vi "Auto2备份.vi"() -> ()   [LabVIEW 2020]
uses:
  Global_Variable/Global.vi
  Libraries/S7/S7.lvlib
  Global_Variable/A180648.vi
  <vilib>/ptbypt/NI_PtbyPt.lvlib
  <userlib>/_MGI/1D Array/MGI Average/MGI Average (DBL[][]).vi
panel:
  out "初始角度":dbl
  out "T1-T2_135°":dbl
  out "T1-T2_225°":dbl
  out "T1-T2_315°":dbl
  out "T1-T2_360°":dbl
  out "T1-T2_270°":dbl
  out "T1-T2_180°":dbl
  out "T1-T2_45°":dbl
  out "T1-T2_90°":dbl
  out "初始化 3":bool[](array[boolean])
  out "动优化态前":cluster{dbl[], dbl[]}[](graph)
  in  "initialize 2":bool caption="初始化"
  in  "initialize":bool caption="初始化"
  out "vRES_cCW":cluster{dbl[], dbl[]}
  out "VRES_cW":cluster{dbl[], dbl[]}
  out "初始化 2":bool[](array[boolean])
  in  "选项卡控件":enum32{"工位二程序复检", "工位二动态复检"}(tab)
  out "传感器复检":cluster{dbl[], dbl[]}[](graph)
  out "动优化态":cluster{dbl[], dbl[]}[](graph)
  in  "请启动":bool
  out "Vres_45°":dbl format="%#.6f"
  out "Vres_135°":dbl format="%#.6f"
  out "Vres_225°":dbl format="%#.6f"
  out "Vres_315°":dbl format="%#.6f"
  out "Vres_360°":dbl format="%#.6f"
  out "Vres_270°":dbl format="%#.6f"
  out "Vres_180°":dbl format="%#.6f"
  out "Vres_90°":dbl format="%#.6f"
  out "S_CCw":dbl[](array[numeric]) caption="数据" format="%0.6f"
  out "P_CCw":dbl[](array[numeric]) caption="数据" format="%0.6f"
  out "S_CW":dbl[](array[numeric]) caption="数据" format="%0.6f"
  out "P_CW":dbl[](array[numeric]) caption="数据" format="%0.6f"
  out "T1_CCw":dbl[](array[numeric]) caption="数据" format="%0.2f"
  out "T2_CCw":dbl[](array[numeric]) caption="数据" format="%0.2f"
  out "T2_CW":dbl[](array[numeric]) caption="数据" format="%0.2f"
  out "T1_CW":dbl[](array[numeric]) caption="数据" format="%0.2f"
  out "初始化":bool[](array[boolean])
  out "SENSOR":T1
  in  "判定结果":bool[][](array[boolean])=[[TRUE]]
  in  "STEP":string
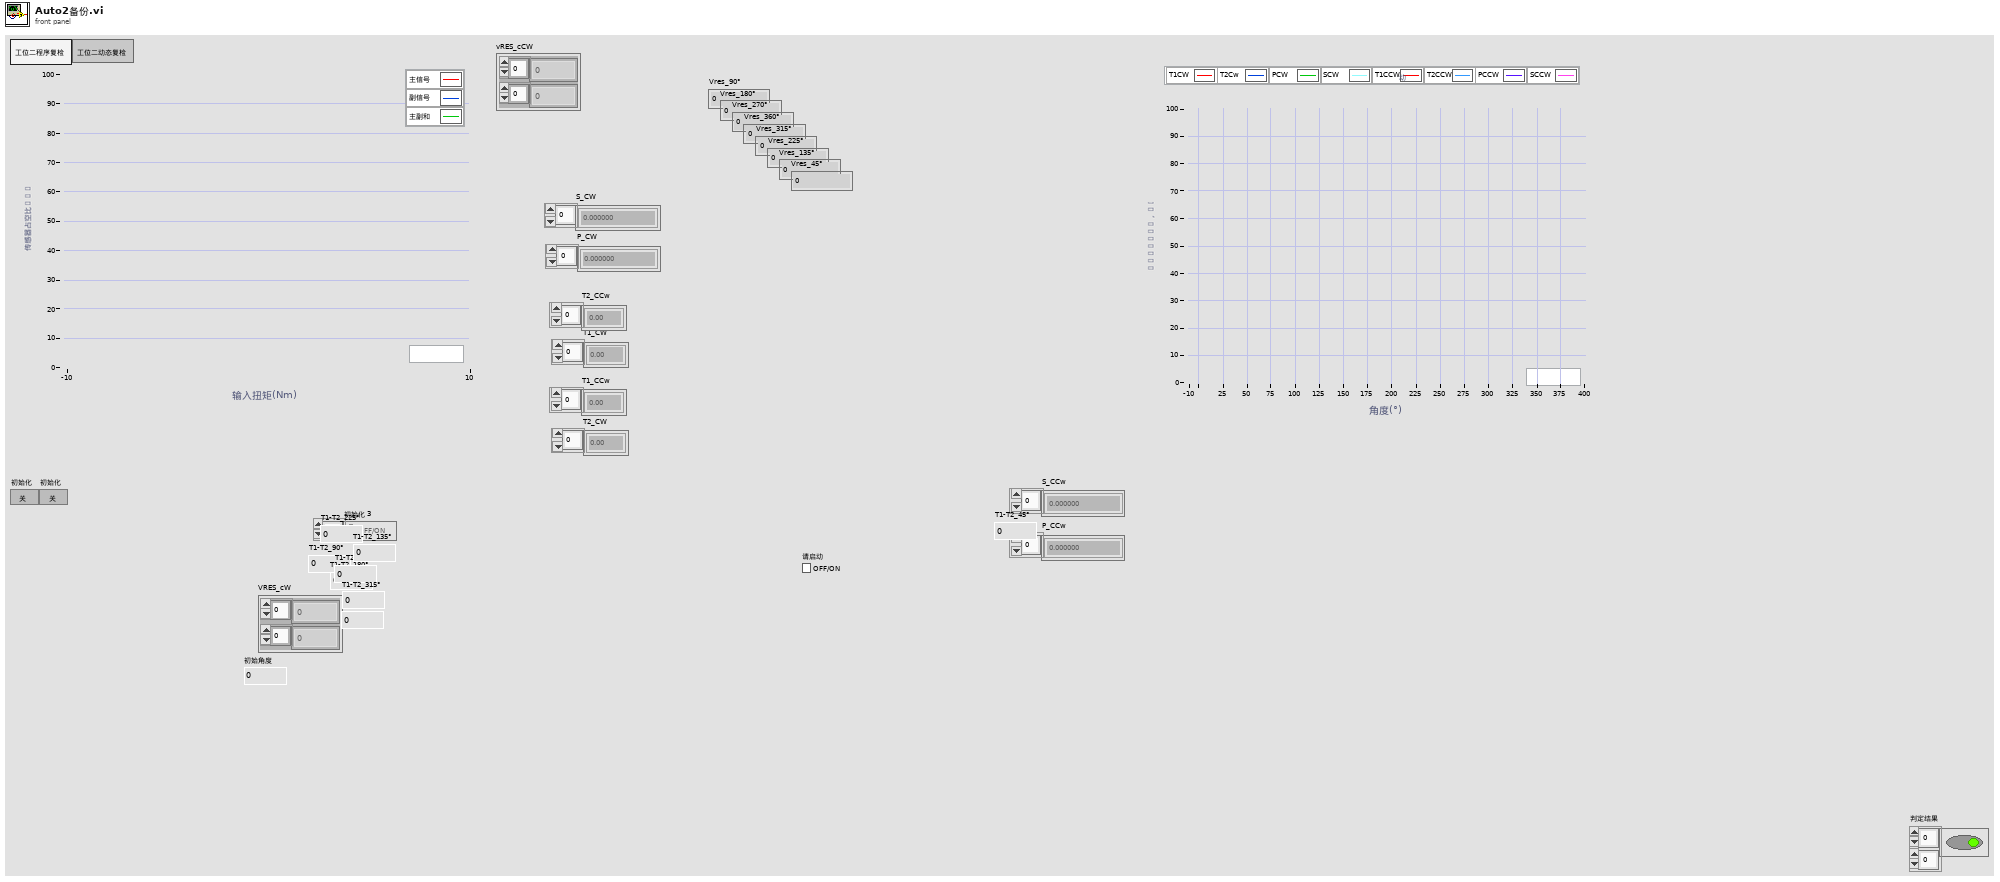
[diagram p1: front panel]
types:
  T1 = cluster{"hSENSOR":i32, "hASIC_T1":i32, "hASIC_T2":i32, "hASIC_P":i32, "hASIC_S":i32}
  T2 = typedef "检测CTR.xctl/检测CTR数据.ctl" = enum16{"Idle", "Runing", "Pass", "Faild", "Skip"}
  T3 = enum32{"Invalid", "Standard", "Closed", "Hidden", "Minimized", "Maximized"}
  T4 = enum16{"Idle", "Runing", "Pass", "Faild", "Skip"}
  T5 = enum16{"open", "replace", "create", "open or create", "replace or create", "replace or create with confirmation"}
  T6 = cluster{"工位一驱动伺服位移":sgl, "工位二驱动伺服位移":sgl, "工位一移载伺服位移":sgl, "工位二移载伺服位移":sgl, "工位一编码器位移":sgl, "工位二编码器位移":sgl, "工位一扭矩":sgl, "工位二扭矩":sgl}
  T7 = cluster{"主副信号和MAX":cluster{"单位":string, "下限":dbl, "上限":dbl}, "主副信号和MIN":cluster{"单位":string, "下限":dbl, "上限":dbl}, "主信号线性误差":cluster{"单位":string, "下限":dbl, "上限":dbl}, "副信号线性误差":cluster{"单位":string, "下限":dbl, "上限":dbl}, "主信号MAX":cluster{"单位":string, "下限":dbl, "上限":dbl}, "主信号MIN":cluster{"单位":string, "下限":dbl, "上限":dbl}, "副信号MAX":cluster{"单位":string, "下限":dbl, "上限":dbl}, "副信号MIN":cluster{"单位":string, "下限":dbl, "上限":dbl}, "中心偏移量":cluster{"单位":string, "下限":dbl, "上限":dbl}, "定点设置":cluster{"单位":string, "下限":dbl, "上限":dbl}, "定点左侧主信号":cluster{"单位":string, "下限":dbl, "上限":dbl}, "定点左侧副信号":cluster{"单位":string, "下限":dbl, "上限":dbl}, "定点右侧主信号":cluster{"单位":string, "下限":dbl, "上限":dbl}, "定点右侧副信号":cluster{"单位":string, "下限":dbl, "上限":dbl}, "监测点1左滞后":cluster{"单位":string, "下限":dbl, "上限":dbl}, "监测点1右滞后":cluster{"单位":string, "下限":dbl, "上限":dbl}, "监测点2左滞后":cluster{"单位":string, "下限":dbl, "上限":dbl}, "监测点2右滞后":cluster{"单位":string, "下限":dbl, "上限":dbl}, "监测点3左滞后":cluster{"单位":string, "下限":dbl, "上限":dbl}, "监测点3右滞后":cluster{"单位":string, "下限":dbl, "上限":dbl}}
  T8 = cluster{"复检速度":dbl, "换向扭矩":dbl, "判定范围下限":dbl, "判定范围上限":dbl, "滞后监测点1":dbl, "滞后监测点2":dbl, "滞后监测点3":dbl}
  T9 = cluster{"动优化态":cluster{dbl[], dbl[]}[], "动优化态前":cluster{dbl[], dbl[]}[], "传感器复检":cluster{dbl[], dbl[]}[]}
  T10 = typedef "lveventtype.ctl" = enum32{"Null", "Timeout", "Annotation Menu Selection", "Annotation Menu Selection?", "App Instance Close", "App Instance Close?", "Autoscale Range Change", "Bookmark Info Change", "Cell Edit", "Cell Edit?", "Cursor Grab", "Cursor Grab?", "Cursor Menu Selection", "Cursor Menu Selection?", "Cursor Move", "Cursor Release", "Data Change", "Direction Change", "Display State Change", "Drag Ended", "Drag Enter", "Drag Leave", "Drag Over", "Drag Source Update", "Drag Starting", "Drag Starting?", "Drop", "Exec State Change", "Key Down", "Key Down?", "Key Repeat", "Key Repeat?", "Key Up", "Listbox Double Click", "Menu Activation?", "Menu Selection (App)", "Menu Selection? (App)", "Menu Selection (User)", "Mouse Down", "Mouse Down?", "Mouse Enter", "Mouse Leave", "Mouse Move", "Mouse Up", "Mouse Wheel", "NI Security User Change (App)", "Pane Size", "Panel Close", "Panel Close?", "Panel Resize", "Plot Attribute Change", "Scale Range Change", "Shortcut Menu Activation?", "Shortcut Menu Selection (App)", "Shortcut Menu Selection? (App)", "Shortcut Menu Selection (User)", "Tree Double Click", "Tree Drag", "Tree Drag?", "Tree Drop", "Tree Drop?", "Tree Item Close", "Tree Item Close?", "Tree Item Open", "Tree Item Open?", "User Event", "Value Change"}
  T11 = typedef "LVPoint32TypeDef.ctl" = cluster{"Horizontal":i32, "Vertical":i32}
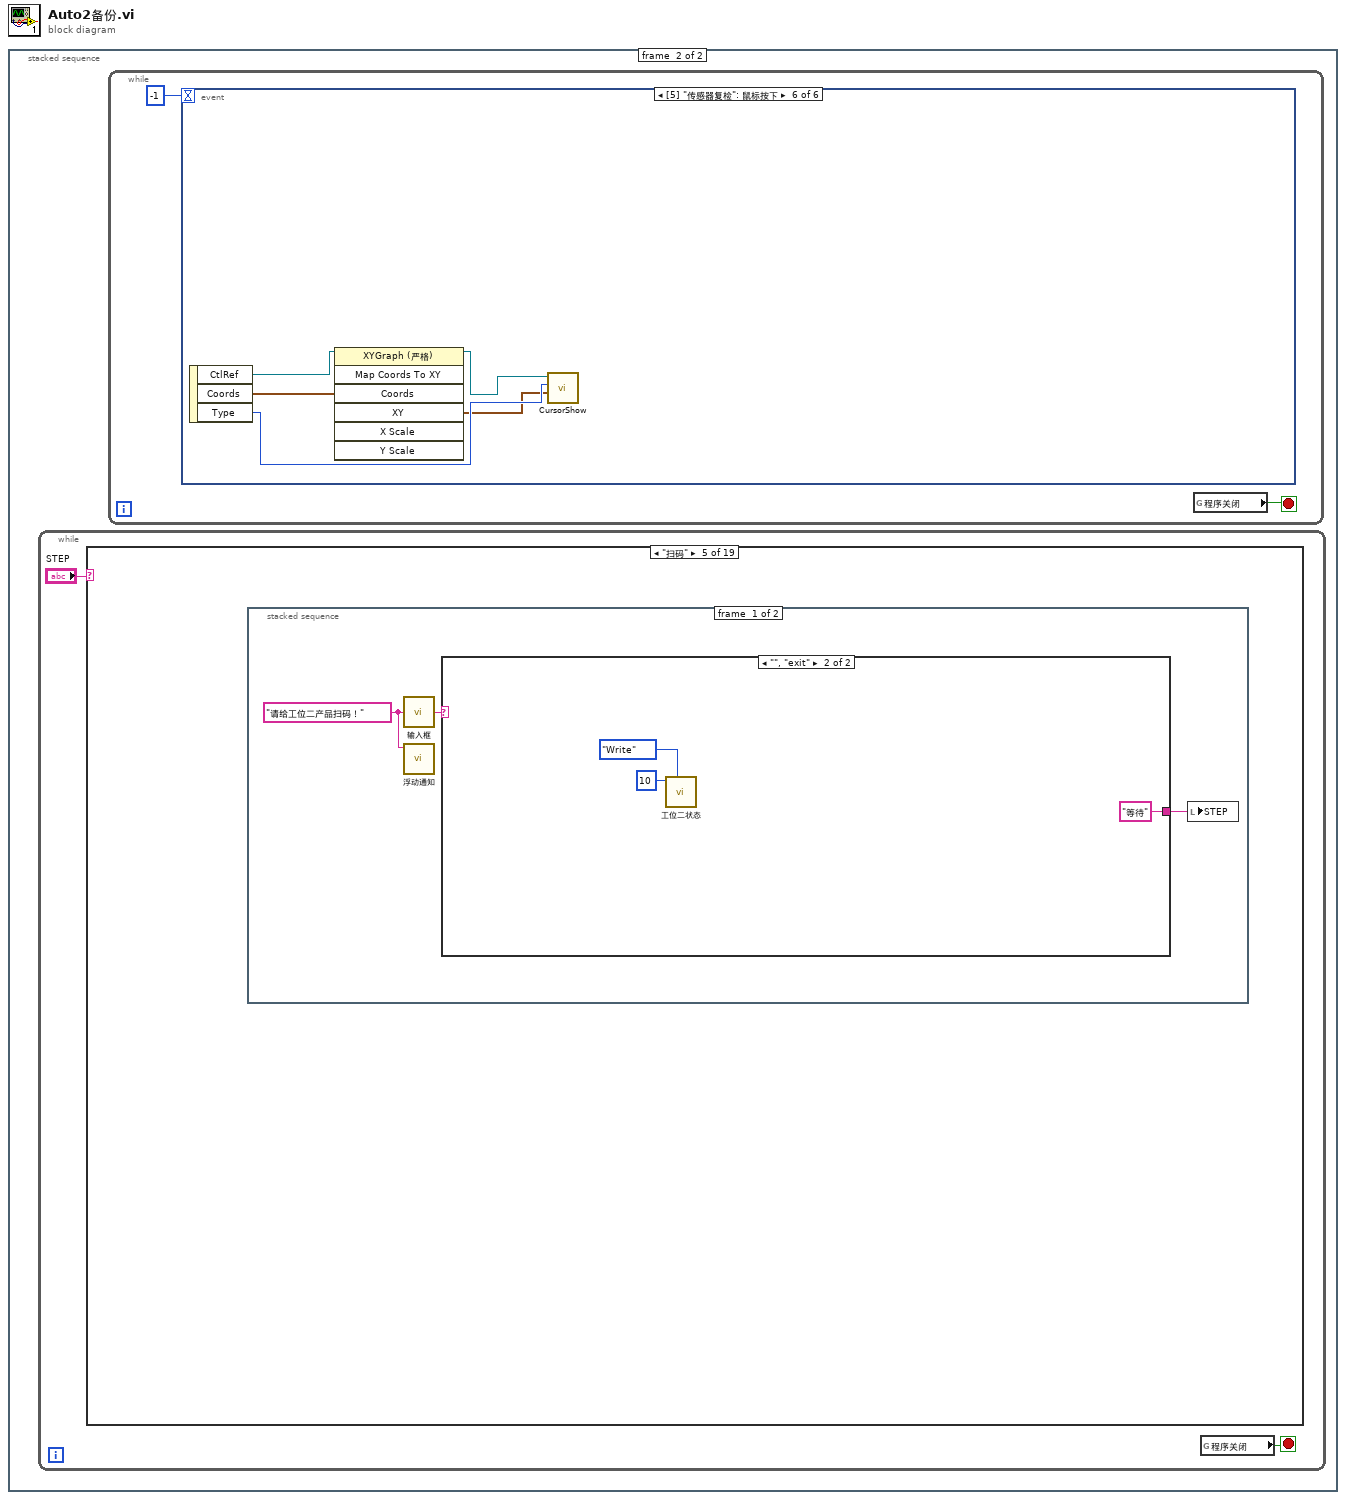
[diagram p0: block diagram]
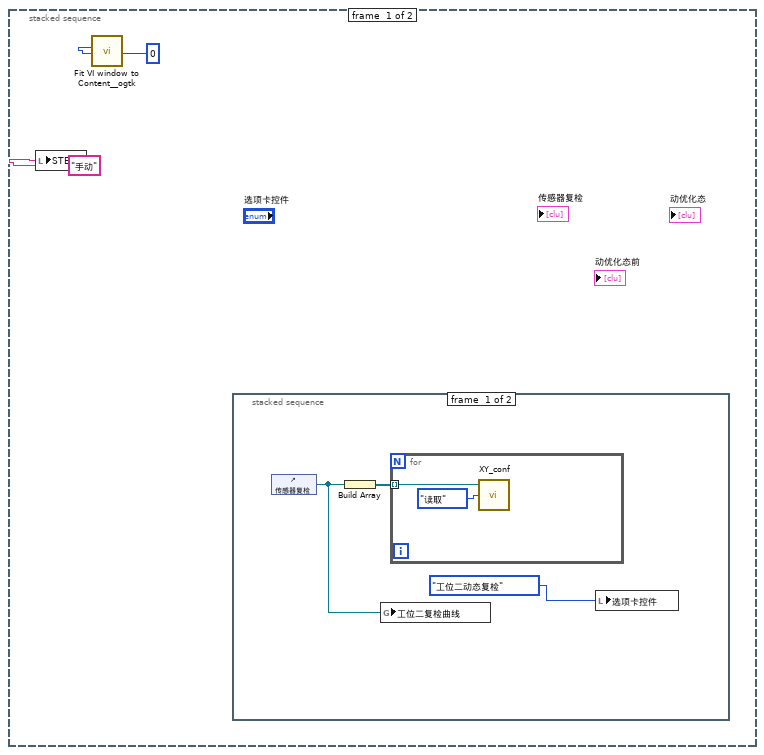
[diagram p2: hidden frame]
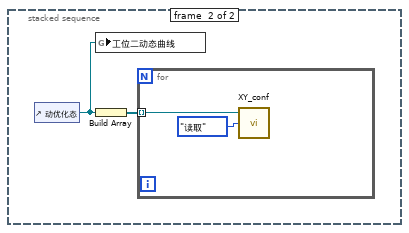
[diagram p3: hidden frame]
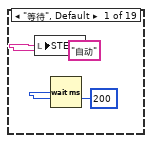
[diagram p4: hidden frame]
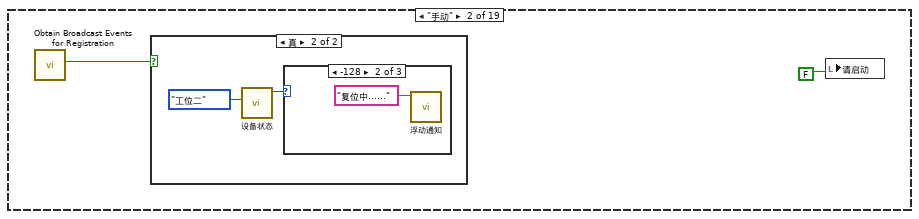
[diagram p5: hidden frame]
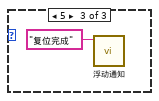
[diagram p8: hidden frame]
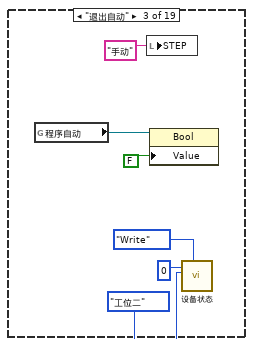
[diagram p9: hidden frame]
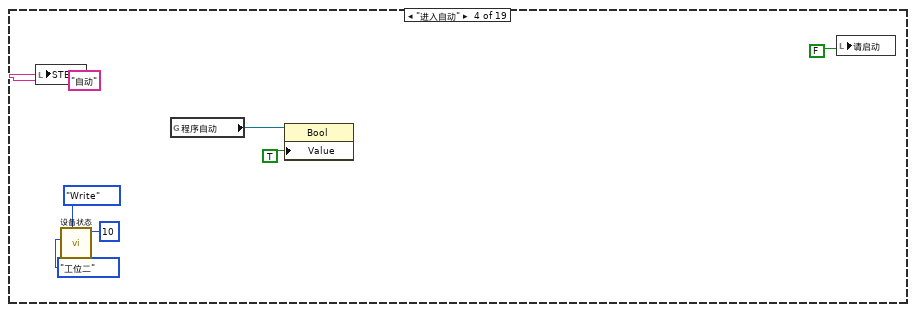
[diagram p10: hidden frame]
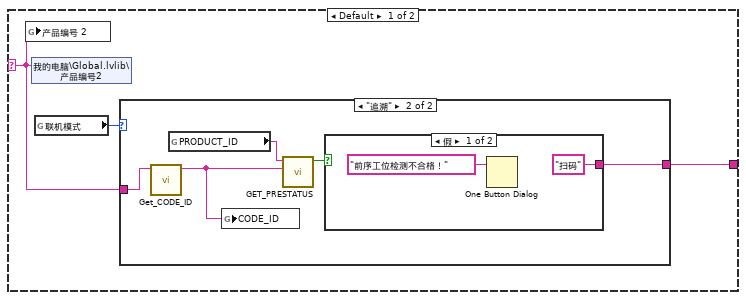
[diagram p11: hidden frame]
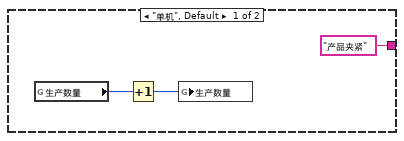
[diagram p12: hidden frame]
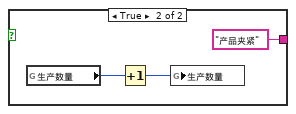
[diagram p13: hidden frame]
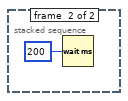
[diagram p14: hidden frame]
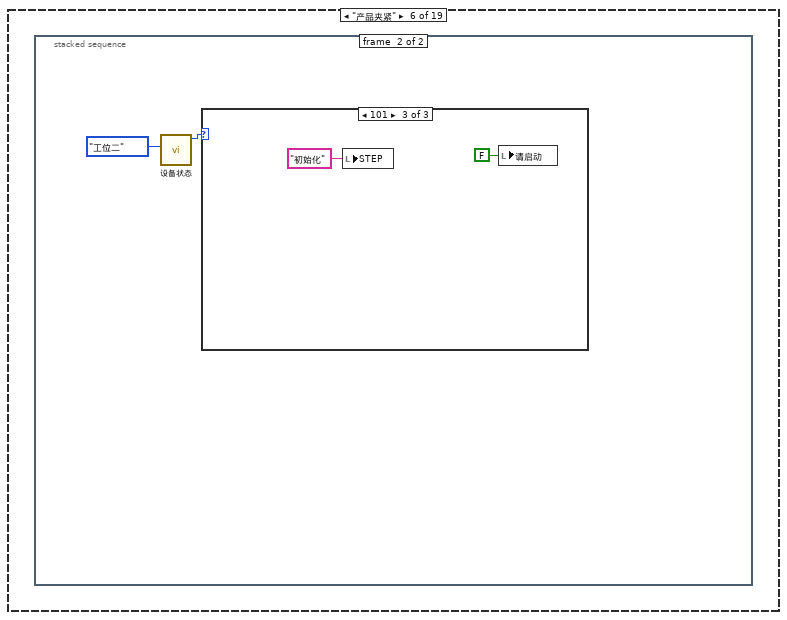
[diagram p15: hidden frame]
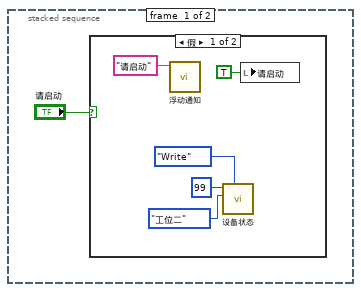
[diagram p16: hidden frame]
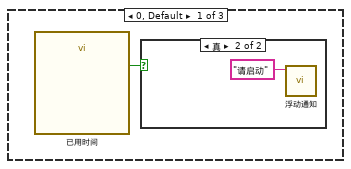
[diagram p18: hidden frame]
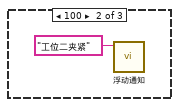
[diagram p20: hidden frame]
diagram:
  n1 = stacked-sequence {
    frame #0 {
      n2 = local write "STEP"("手动" ("STEP")) -> ()
      n3 = call <userlib>:"Fit VI window to Content__ogtk.vi"("border spacing (2 px)"=0) -> ()  [unwired: 5 in, 2 out]
      n4 = stacked-sequence {
        frame #0 {
          n5 = control-ref of="传感器复检"() -> (w4:refnum<vi>)
          n6 = Build Array(w4) -> (w5:refnum<vi>[])
          n7 = global write "A180648.vi" "工位二复检曲线"(w4) -> ()
          n8 = for {
            tunnel: w5 -> [w6] mode=indexing
            n9 = call "XY_conf.vi"("方式"=enum16{"写入", "读取"}."读取", "XY图引用"=w6) -> ()  [unwired: 3 in, 1 out]
          }
          n10 = local write "选项卡控件"(enum32{"工位二程序复检", "工位二动态复检"}."工位二动态复检" ("选项卡控件")) -> ()
        }
        frame #1 {
          n11 = control-ref of="动优化态"() -> (w9:refnum<vi>)
          n12 = global write "A180648.vi" "工位二动态曲线"(w9) -> ()
          n13 = Build Array(w9) -> (w8:refnum<vi>[])
          n14 = for {
            tunnel: w8 -> [w10] mode=indexing
            n15 = call "XY_conf.vi"("方式"=enum16{"写入", "读取"}."读取", "XY图引用"=w10) -> ()  [unwired: 3 in, 1 out]
          }
        }
      }
    }
    frame #1 {
      n16 = while {
        stop <- w13 stop-if-true
        n17 = case shown="\"扫码\"" "STEP" {
          frame "等待", Default {
            n18 = local write "STEP"("自动" ("STEP")) -> ()
            n19 = Wait (ms)(milliseconds to wait=u32 200 ("等待时间（毫秒）")) -> ()  [unwired: 1 out]
          }
          frame "手动" {
            n20 = call "Obtain Broadcast Events for Registration.vi"() -> ("Already running?"=w17:bool)  [unwired: 9 in, 2 out]
            n21 = case shown="真" w17 {
              frame False {
              }
              frame True {
                n22 = call "设备状态.vi"("工位"=enum16{"工位一", "工位二"}."工位二") -> ("Status_Read"=w19:i16)  [unwired: 10 in]
                n23 = case shown="-128" w19 {
                  frame 0, Default {
                  }
                  frame -128 {
                    n24 = call "浮动通知.vi"("通知内容"="复位中……" ("Status")) -> ()  [unwired: 11 in]
                  }
                  frame 5 {
                    n25 = call "浮动通知.vi"("通知内容"="复位完成" ("Status")) -> ()  [unwired: 11 in]
                  }
                }
              }
            }
            n26 = local write "请启动"(FALSE ("请启动")) -> ()
          }
          frame "退出自动" {
            n27 = global read "Global.vi" "程序自动"() -> (w24:refnum<vi>)
            n28 = local write "STEP"("手动" ("STEP")) -> ()
            n29 = property class="Bool"(reference=w24, "Value"=FALSE) -> ()  [unwired: 1 in, 2 out]
            n30 = call "设备状态.vi"("枚举"=enum16{"Read", "Write"}."Write", "工位"=enum16{"工位一", "工位二"}."工位二", "Status_Write"=i16 0) -> ()  [unwired: 8 in, 1 out]
          }
          frame "进入自动" {
            n31 = local write "STEP"("自动" ("STEP")) -> ()
            n32 = call "设备状态.vi"("枚举"=enum16{"Read", "Write"}."Write", "工位"=enum16{"工位一", "工位二"}."工位二", "Status_Write"=i16 10) -> ()  [unwired: 8 in, 1 out]
            n33 = global read "Global.vi" "程序自动"() -> (w33:refnum<vi>)
            n34 = property class="Bool"(reference=w33, "Value"=TRUE) -> ()  [unwired: 1 in, 2 out]
            n35 = local write "请启动"(FALSE ("请启动")) -> ()
          }
          frame "扫码" {
            n36 = stacked-sequence {
              frame #0 {
                w36 = "请给工位二产品扫码！" ("提示信息")
                n37 = call "输入框.vi"("提示信息"=w36) -> ("条形码输出"=w37:string)
                n38 = call "浮动通知.vi"("通知内容"=w36) -> ()  [unwired: 11 in]
                n39 = case shown="\"\", \"exit\"" w37 {
                  selector: w37 -> [w38 _]
                  tunnel: [w40 "等待" ("State(s) in Front (\"\")")] -> w35
                  frame Default {
                    n40 = global write "Global.vi" "产品编号 2"(w38) -> ()
                    n41 = shared-variable "我的电脑\\Global.lvlib\\产品编号2"(w38) -> ()  [unwired: 1 in, 1 out]
                    n42 = global read "Global.vi" "联机模式"() -> (w39:enum16{"单机", "追溯"})
                    n43 = case shown="\"追溯\"" w39 {
                      tunnel: ["产品夹紧" ("State(s) in Front (\"\")") w48] -> w40
                      tunnel: w38 -> [_ w45]
                      frame "单机", Default {
                        n44 = global read "Global.vi" "生产数量"() -> (w41:i32)
                        n45 = Increment(x=w41) -> (x+1=w42:i32)
                        n46 = global write "Global.vi" "生产数量"(w42) -> ()
                      }
                      frame "追溯" {
                        n47 = call "Get_CODE_ID.vi"("CODE_MAIN"=w45) -> ("CODE_ID"=w44:string)  [unwired: 10 in]
                        n48 = global read "追溯Global.vi" "PRODUCT_ID"() -> (w47:string)
                        n49 = global write "追溯Global.vi" "CODE_ID"(w44) -> ()
                        n50 = call "GET_PRESTATUS.vi"("CODE_ID"=w44, "PRODUCT_ID"=w47) -> ("OK?"=w46:bool)  [unwired: 9 in]
                        n51 = case shown="假" w46 {
                          tunnel: ["扫码" ("State(s) in Front (\"\")") "产品夹紧" ("State(s) in Front (\"\")")] -> w48
                          frame False {
                            n52 = One Button Dialog(message="前序工位检测不合格！" ("消息")) -> ()  [unwired: 1 in, 1 out]
                          }
                          frame True {
                            n53 = global read "Global.vi" "生产数量"() -> (w51:i32)
                            n54 = Increment(x=w51) -> (x+1=w52:i32)
                            n55 = global write "Global.vi" "生产数量"(w52) -> ()
                          }
                        }
                      }
                    }
                  }
                  frame "", "exit" {
                    n56 = call "工位二状态.vi"("枚举"=enum16{"Read", "Write"}."Write", "Status_Write"=i16 10) -> ()  [unwired: 9 in, 1 out]
                  }
                }
                n57 = local write "STEP"(w35) -> ()
              }
              frame #1 {
                n58 = Wait (ms)(milliseconds to wait=u32 200 ("等待时间（毫秒）")) -> ()  [unwired: 1 out]
              }
            }
          }
          frame "产品夹紧" {
            n59 = stacked-sequence {
              frame #0 {
                n60 = case shown="假" "请启动" {
                  frame False {
                    n61 = call "浮动通知.vi"("通知内容"="请启动" ("Status")) -> ()  [unwired: 11 in]
                    n62 = call "设备状态.vi"("枚举"=enum16{"Read", "Write"}."Write", "工位"=enum16{"工位一", "工位二"}."工位二", "Status_Write"=i16 99) -> ()  [unwired: 8 in, 1 out]
                    n63 = local write "请启动"(TRUE ("请启动")) -> ()
                  }
                  frame True {
                  }
                }
              }
              frame #1 {
                n64 = call "设备状态.vi"("工位"=enum16{"工位一", "工位二"}."工位二") -> ("Status_Read"=w64:i16)  [unwired: 10 in]
                n65 = case shown="101" w64 {
                  frame 0, Default {
                    n66 = call "已用时间"() -> ("Time has Elapsed"=w66:bool)  [unwired: 12 in, 7 out]
                    n67 = case shown="真" w66 {
                      frame False {
                      }
                      frame True {
                        n68 = call "浮动通知.vi"("通知内容"="请启动" ("Status")) -> ()  [unwired: 11 in]
                      }
                    }
                  }
                  frame 100 {
                    n69 = call "浮动通知.vi"("通知内容"="工位二夹紧" ("Status")) -> ()  [unwired: 11 in]
                  }
                  frame 101 {
                    n70 = local write "STEP"("初始化") -> ()
                    n71 = local write "请启动"(FALSE ("请启动")) -> ()
                  }
                }
              }
            }
          }
          frame "套输入轴" {
            n72 = global read "Global.vi" "复检2引用句柄"() -> (w80)
            n73 = global read "Global.vi" "动态优化 2"() -> (w77)
            n74 = property class="检测CTR"(reference=w77) -> ("Value"=w78:variant)  [unwired: 1 in, 2 out]
            n75 = property class="检测CTR"(reference=w80) -> ("Value"=w79:variant)  [unwired: 1 in, 2 out]
            n76 = Variant To Data(type=检测CTR数据."Idle" ("Data"), Variant=w78) -> (data=w76:T2)  [unwired: 1 in, 1 out]
            n77 = Variant To Data(type=检测CTR数据."Idle" ("Data"), Variant=w79) -> (data=w81:T2)  [unwired: 1 in, 1 out]
            n78 = Equal?(x=w76, y=检测CTR数据."Skip" ("Data")) -> (x = y?=w82:bool)
            n79 = Equal?(x=w81, y=检测CTR数据."Skip" ("Data")) -> (x = y?=w83:bool)
            n80 = And(x=w82, y=w83) -> (x .and. y?=w71:bool)
            n81 = case shown="假" w71 {
              frame False {
                n82 = stacked-sequence {
                  frame #0 {
                    n83 = call "浮动通知.vi"("通知内容"="工位二产品套输入轴" ("Status")) -> ()  [unwired: 11 in]
                    n84 = call "设备状态.vi"("枚举"=enum16{"Read", "Write"}."Write", "工位"=enum16{"工位一", "工位二"}."工位二", "Status_Write"=i16 112) -> ()  [unwired: 8 in, 1 out]
                    n85 = vi-ref "T1T2占空比2.vi"() -> (w87:refnum<vi>)
                    n86 = call "CallVI.vi"("VI引用"=w87, "状态"=T3."Hidden") -> ()  [unwired: 12 in, 2 out]
                    n87 = vi-ref "PS采集2.vi"() -> (w84:refnum<vi>)
                    n88 = call "CallVI.vi"("VI引用"=w84, "状态"=T3."Hidden") -> ()  [unwired: 12 in, 2 out]
                  }
                  frame #1 {
                    n89 = while {
                      stop <- w92 stop-if-true
                      n90 = call "设备状态.vi"("工位"=enum16{"工位一", "工位二"}."工位二") -> ("Status_Read"=w93:i16)  [unwired: 10 in]
                      n91 = case shown="113" w93 {
                        tunnel: [w95 TRUE] -> w92
                        frame 0, Default {
                          n92 = call "套输入轴时间"() -> ("Time has Elapsed"=w96:bool)  [unwired: 12 in, 7 out]
                          n93 = case shown="真" w96 {
                            tunnel: [FALSE TRUE] -> w95
                            frame False {
                            }
                            frame True {
                              n94 = call "浮动通知.vi"("通知内容"="工位二产品套输入轴超时" ("Status")) -> ()  [unwired: 11 in]
                            }
                          }
                        }
                        frame 113 {
                          n95 = local write "STEP"("动态优化") -> ()
                        }
                      }
                    }
                  }
                }
              }
              frame True {
                n96 = local write "STEP"("程序固化" ("STEP")) -> ()
              }
            }
          }
          frame "套输出轴" {
            n97 = global read "Global.vi" "复检2引用句柄"() -> (w107)
            n98 = property class="检测CTR"(reference=w107) -> ("Value"=w106:variant)  [unwired: 1 in, 2 out]
            n99 = Variant To Data(type=检测CTR数据."Idle" ("Data"), Variant=w106) -> (data=w108:T2)  [unwired: 1 in, 1 out]
            n100 = Equal?(x=w108, y=检测CTR数据."Skip" ("Data")) -> (x = y?=w103:bool)
            n101 = case shown="假" w103 {
              frame False {
                n102 = stacked-sequence {
                  frame #0 {
                    n103 = call "设备状态.vi"("枚举"=enum16{"Read", "Write"}."Write", "工位"=enum16{"工位一", "工位二"}."工位一", "Status_Write"=i16 108) -> ()  [unwired: 8 in, 1 out]
                    n104 = call "浮动通知.vi"("通知内容"="工位一产品套输出轴" ("Status")) -> ()  [unwired: 11 in]
                  }
                  frame #1 {
                    n105 = while {
                      stop <- w113 stop-if-true
                      n106 = call "设备状态.vi"("工位"=enum16{"工位一", "工位二"}."工位二") -> ("Status_Read"=w114:i16)  [unwired: 10 in]
                      n107 = case shown="109" w114 {
                        tunnel: [w116 TRUE] -> w113
                        frame 0, Default {
                          n108 = call "套输出轴时间"() -> ("Time has Elapsed"=w117:bool)  [unwired: 12 in, 7 out]
                          n109 = case shown="真" w117 {
                            tunnel: [FALSE TRUE] -> w116
                            frame False {
                            }
                            frame True {
                              n110 = call "浮动通知.vi"("通知内容"="工位二产品套输出轴超时" ("Status")) -> ()  [unwired: 11 in]
                            }
                          }
                        }
                        frame 109 {
                          n111 = call "传感器数据.vi"() -> ("传感器读数"=w122:T6)  [unwired: 11 in]
                          n112 = local write "STEP"("程序复检") -> ()
                          n113 = Unbundle By Name(w122) -> ("工位二驱动伺服位移"=→"初始角度":sgl)
                        }
                      }
                    }
                  }
                }
              }
              frame True {
                n114 = local write "STEP"("程序固化" ("STEP")) -> ()
              }
            }
          }
          frame "初始化" {
            n115 = stacked-sequence {
              frame #0 {
                w128 = cluster{dbl[], dbl[]} {[], []} ("vRES_cCW")
                n116 = disable-structure shown="禁用" {
                  frame Disabled {
                    n117 = global write "Global.vi" "计时开始"(TRUE ("计时开始")) -> ()
                  }
                  frame Enabled {
                  }
                }
                n118 = global write "Global.vi" "IO_Stop"(TRUE ("IO_Stop")) -> ()
                n119 = global write "Global.vi" "工位二占空比采集"(FALSE ("工位二占空比采集")) -> ()
                n120 = global write "Global.vi" "P/S采集 2"(FALSE ("工位二占空比采集")) -> ()
                n121 = local write "判定结果"(bool[][] [] ("判定结果")) -> ()
                n122 = global write "Global.vi" "动态优化完成"(FALSE ("动态优化完成")) -> ()
                n123 = local write "vRES_cCW"(w128) -> ()
                n124 = local write "VRES_cW"(w128) -> ()
                n125 = local write "选项卡控件"(enum32{"工位二程序复检", "工位二动态复检"}."工位二动态复检" ("选项卡控件")) -> ()
              }
              frame #1 {
                w139 = dbl[] [] ("S_CCw")
                w140 = dbl[] [] ("T1_cw")
                n126 = local write "T1_CW"(w140) -> ()
                n127 = local write "T2_CW"(w140) -> ()
                n128 = local write "P_CW"(w140) -> ()
                n129 = local write "P_CCw"(w140) -> ()
                n130 = for {
                  N: 12 -> [_]
                  tunnel: [cluster{dbl[], dbl[]} {[], []}] -> w138 mode=indexing
                }
                n131 = local write "传感器复检"(w138) -> ()
                n132 = local write "S_CCw"(w139) -> ()
                n133 = local write "S_CW"(w139) -> ()
                n134 = local write "T1_CCw"(w139) -> ()
                n135 = local write "T2_CCw"(w139) -> ()
                n136 = for {
                  N: 8 -> [_]
                  tunnel: [cluster{dbl[], dbl[]} {[], []}] -> w136 mode=indexing
                }
                n137 = for {
                  N: 8 -> [_]
                  tunnel: [cluster{dbl[], dbl[]} {[], []}] -> w135 mode=indexing
                }
                n138 = local write "动优化态前"(w135) -> ()
                n139 = local write "动优化态"(w136) -> ()
              }
              frame #2 {
                n140 = global read "Global.vi" "Result 2"() -> (w156)
                n141 = property class="Tbl"(reference=w156, "Value"=string[][] []) -> (reference out=w157:refnum<vi>, error out=w158:errorcluster)  [unwired: 1 in]
                n142 = property class="Tbl"(reference=w157, error in=w158, "Row Headers[]"=string[] [] ("列首字符串[]")) -> ()  [unwired: 2 out]
                n143 = Initialize Array(TRUE, 12 ("维数大小")) -> (→"初始化":bool[])
                n144 = Initialize Array(TRUE, 8 ("维数大小")) -> (→"初始化 2":bool[])
                n145 = Initialize Array(TRUE, 8 ("维数大小")) -> (→"初始化 3":bool[])
              }
              frame #3 {
                n146 = global read "Global.vi" "静态标定2引用句柄"() -> (w163)
                n147 = global read "Global.vi" "程序固化2引用句柄"() -> (w162)
                n148 = global read "Global.vi" "复检2引用句柄"() -> (w161)
                n149 = global read "Global.vi" "动态优化 2"() -> (w159)
                n150 = Build Array(w163, w162, w161, w159) -> (w160:void[])
                n151 = for {
                  tunnel: w160 -> [w173] mode=indexing
                  n152 = property class="检测CTR"(reference=w173) -> (reference out=w172:refnum<vi>, "Value"=w171:variant)  [unwired: 1 in, 1 out]
                  n153 = Variant To Data(type=检测CTR数据."Idle" ("Data"), Variant=w171) -> (data=w169:T2)  [unwired: 1 in, 1 out]
                  n154 = Equal?(x=w169, y=检测CTR数据."Skip" ("Data")) -> (x = y?=w167:bool)
                  n155 = Select(t=检测CTR数据."Skip" ("Data"), s=w167, f=检测CTR数据."Idle" ("Data")) -> (s? t:f=w164:T2)
                  n156 = property class="检测CTR"(reference=w172, "Value"=w164) -> ()  [unwired: 1 in, 2 out]
                }
              }
              frame #4 {
                n157 = local write "STEP"("静态标定" ("STEP")) -> ()
              }
            }
          }
          frame "静态标定" {
            n158 = global read "Global.vi" "静态标定2引用句柄"() -> (w179)
            n159 = property class="检测CTR"(reference=w179) -> ("Value"=w178:variant)  [unwired: 1 in, 2 out]
            n160 = Variant To Data(type=检测CTR数据."Idle" ("Data"), Variant=w178) -> (data=w180:T2)  [unwired: 1 in, 1 out]
            n161 = Equal?(x=w180, y=检测CTR数据."Skip" ("Data")) -> (x = y?=w175:bool)
            n162 = case shown="假" w175 {
              frame False {
                n163 = stacked-sequence {
                  tunnel: [_ _ w189] -> w181
                  frame #0 {
                    n164 = call "InitPGI.vi"("DeviceNumber"=2) -> ("SENSOR"=w183:T1, "error out"=w184:errorcluster)  [unwired: 13 in]
                    "SENSOR" <- w183
                    n165 = call "InitProduct.vi"("SENSOR"=w183, "error in (no error)"=w184) -> ()  [unwired: 12 in, 2 out]
                  }
                  frame #1 {
                    n166 = global read "Global.vi" "静态标定2引用句柄"() -> (w186)
                    n167 = call "浮动通知.vi"("通知内容"="静态标定" ("Status")) -> ()  [unwired: 11 in]
                    n168 = property class="检测CTR"(reference=w186, "Value"=T4."Runing" ("值")) -> ()  [unwired: 1 in, 2 out]
                  }
                  frame #2 {
                    n169 = flat-sequence {
                      frame #0 {
                        n170 = call "采集切换2.vi"("切换"=TRUE) -> ()  [unwired: 10 in, 1 out]
                      }
                      frame #1 {
                        n171 = call "Wait1.vi"("Wait（150ms）"=u32 500) -> ()  [unwired: 2 in, 1 out]
                      }
                      frame #2 {
                        n172 = call "采集切换2.vi"("切换"=FALSE) -> ()  [unwired: 10 in, 1 out]
                      }
                      frame #3 {
                        n173 = call "采集切换2.vi"("切换"=TRUE) -> ()  [unwired: 10 in, 1 out]
                      }
                      frame #4 {
                        n174 = call "采集切换2.vi"("切换"=FALSE) -> ()  [unwired: 10 in, 1 out]
                      }
                      frame #5 {
                        n175 = call "采集切换2.vi"("切换"=TRUE) -> ()  [unwired: 10 in, 1 out]
                      }
                      frame #6 {
                        n176 = call "Wait1.vi"("Wait（150ms）"=u32 200) -> ()  [unwired: 2 in, 1 out]
                      }
                      frame #7 {
                        n177 = call "采集切换2.vi"("切换"=FALSE) -> ()  [unwired: 10 in, 1 out]
                      }
                    }
                    n178 = local read "SENSOR"() -> (w190:T1)
                    n179 = call "StaticCalibration2备份.vi"("SENSOR"=w190) -> ("OK"=w188:bool)  [unwired: 6 in, 8 out]
                    n180 = case shown="真" w188 {
                      tunnel: [w199 "套输入轴"] -> w189
                      frame False {
                        n181 = global read "Global.vi" "静态标定2引用句柄"() -> (w207)
                        n182 = property class="检测CTR"(reference=w207, "Value"=T4."Faild" ("值")) -> ()  [unwired: 1 in, 2 out]
                        n183 = Two Button Dialog(message="静态标定失败\n建议旋转传感器后重新标定\n是否重新标定？" ("消息"), 1:"否" ("F按钮名称（“取消”）"), 2:"是" ("T按钮名称（“确定”）")) -> (T button?=w202:bool)
                        n184 = Select(t="初始化" ("T按钮名称（“确定”）"), s=w202, f="不合格" ("F按钮名称（“取消”）")) -> (s? t:f=w199:string)
                      }
                      frame True {
                        n185 = global read "Global.vi" "静态标定引用句柄"() -> (w212:refnum<vi>)
                        n186 = local read "判定结果"() -> (w208:bool[][])
                        n187 = Build Array (concatenate)(w208, bool[][] [[TRUE, TRUE]] ("判定结果")) -> (w210:bool[][])
                        n188 = local write "判定结果"(w210) -> ()
                        n189 = property class="检测CTR"(reference=w212, "Value"=T4."Pass" ("值")) -> ()  [unwired: 1 in, 2 out]
                      }
                    }
                  }
                }
                n190 = local write "STEP"(w181) -> ()
              }
              frame True {
                n191 = local write "STEP"("套输入轴") -> ()
                n192 = local read "判定结果"() -> (w214:bool[][])
                n193 = Build Array (concatenate)(w214, bool[][] [[FALSE, TRUE], [FALSE, TRUE]] ("判定结果")) -> (w216:bool[][])
                n194 = local write "判定结果"(w216) -> ()
              }
            }
          }
          frame "动态优化" {
            n195 = global read "Global.vi" "动态优化 2"() -> (w222)
            n196 = property class="检测CTR"(reference=w222) -> ("Value"=w221:variant)  [unwired: 1 in, 2 out]
            n197 = Variant To Data(type=检测CTR数据."Idle" ("Data"), Variant=w221) -> (data=w223:T2)  [unwired: 1 in, 1 out]
            n198 = Equal?(x=w223, y=检测CTR数据."Skip" ("Data")) -> (x = y?=w218:bool)
            n199 = case shown="假" w218 {
              frame False {
                n200 = stacked-sequence {
                  frame #0 {
                    n201 = global read "Global.vi" "动态优化 2"() -> (w226)
                    n202 = call "浮动通知.vi"("通知内容"="动态优化" ("Status")) -> ()  [unwired: 11 in]
                    n203 = property class="检测CTR"(reference=w226, "Value"=T4."Runing" ("值")) -> ()  [unwired: 1 in, 2 out]
                  }
                  frame #1 {
                    n204 = global read "Global.vi" "跳过优化"() -> (w228:bool)
                    n205 = case shown="真" w228 {
                      selector: w228 -> [_ w235]
                      tunnel: ["自动" w233] -> w227
                      frame False {
                        n206 = call "设备状态.vi"("枚举"=enum16{"Read", "Write"}."Write", "工位"=enum16{"工位一", "工位二"}."工位二", "Status_Write"=i16 505) -> ()  [unwired: 8 in, 1 out]
                      }
                      frame True {
                        n207 = global read "Global.vi" "动态优化复测"() -> (w234:bool)
                        n208 = global write "Global.vi" "动态优化完成"(w235) -> ()
                        n209 = case shown="假" w234 {
                          tunnel: [w236 "自动"] -> w233
                          frame False {
                            n210 = global read "Global.vi" "8点复测"() -> (w237:bool)
                            n211 = case shown="假" w237 {
                              tunnel: ["复测判定" "复测"] -> w236
                              frame False {
                              }
                              frame True {
                              }
                            }
                          }
                          frame True {
                            n212 = call "设备状态.vi"("枚举"=enum16{"Read", "Write"}."Write", "工位"=enum16{"工位一", "工位二"}."工位一", "Status_Write"=i16 505) -> ()  [unwired: 8 in, 1 out]
                          }
                        }
                      }
                    }
                    n213 = local write "STEP"(w227) -> ()
                  }
                }
              }
              frame True {
                n214 = local write "STEP"("套输出轴") -> ()
                n215 = local read "判定结果"() -> (w245:bool[][])
                n216 = Build Array (concatenate)(w245, bool[][] [[FALSE, TRUE]] ("判定结果")) -> (w246:bool[][])
                n217 = local write "判定结果"(w246) -> ()
              }
            }
          }
          frame "复测" {
            n218 = stacked-sequence {
              frame #0 {
                n219 = Wait (ms)(milliseconds to wait=u32 300 ("等待时间（毫秒）")) -> ()  [unwired: 1 out]
              }
              frame #1 {
                n220 = local write "STEP"("自动") -> ()
                n221 = call "浮动通知.vi"("通知内容"="复测" ("Status")) -> ()  [unwired: 11 in]
                n222 = call "设备状态.vi"("枚举"=enum16{"Read", "Write"}."Write", "工位"=enum16{"工位一", "工位二"}."工位二", "Status_Write"=i16 510) -> ()  [unwired: 8 in, 1 out]
              }
            }
          }
          frame "复测判定" {
            n223 = local read "Vres_90°"() -> (w273:dbl)
            n224 = local read "Vres_180°"() -> (w272:dbl)
            n225 = local read "Vres_270°"() -> (w271:dbl)
            n226 = local read "Vres_360°"() -> (w270:dbl)
            n227 = local read "Vres_315°"() -> (w265:dbl)
            n228 = local read "Vres_225°"() -> (w264:dbl)
            n229 = local read "Vres_135°"() -> (w263:dbl)
            n230 = local read "Vres_45°"() -> (w269:dbl)
            n231 = local read "T1-T2_90°"() -> (w262:dbl)
            n232 = local read "T1-T2_180°"() -> (w261:dbl)
            n233 = local read "T1-T2_270°"() -> (w260:dbl)
            n234 = local read "T1-T2_360°"() -> (w256:dbl)
            n235 = local read "T1-T2_315°"() -> (w257:dbl)
            n236 = local read "T1-T2_225°"() -> (w258:dbl)
            n237 = local read "T1-T2_135°"() -> (w259:dbl)
            n238 = local read "T1-T2_45°"() -> (w268:dbl)
            n239 = Build Array(w273, w272, w271, w270, w265, w264, w263, w269) -> (w254:dbl[])
            n240 = Build Array(w262, w261, w260, w256, w257, w258, w259, w268) -> (w267:dbl[])
            n241 = Absolute Value(x=w267) -> (abs(x)=w266:dbl[])
            n242 = disable-structure shown="禁用" {
              frame Disabled {
                n243 = Two Button Dialog(message="复测失败\n请选择是否继续？" ("消息"), 1:"否" ("F按钮名称（“取消”）"), 2:"是" ("T按钮名称（“确定”）")) -> ()  [unwired: 1 out]
                n244 = case shown="真" {
                  selector: _ -> [_ _]
                  frame False {
                  }
                  frame True {
                    n245 = local write "STEP"("套输出轴" ("T按钮名称（“确定”）")) -> ()
                  }
                }
              }
              frame Enabled {
              }
            }
            n246 = call "动态优化复测判定.vi"("T1-T2"=w266, "Vres"=w254) -> ("结果1"=w255:bool)  [unwired: 9 in]
            n247 = case shown="真" w255 {
              frame False {
                w280 = enum16{"Read", "Write"}."Write" ("枚举")
                w279 = enum16{"工位一", "工位二"}."工位二" ("工位")
                n248 = global read "Global.vi" "动态优化 2"() -> (w287)
                n249 = local read "判定结果"() -> (w283:bool[][])
                n250 = Build Array (concatenate)(w283, bool[][] [[TRUE, FALSE]] ("判定结果")) -> (w284:bool[][])
                n251 = local write "判定结果"(w284) -> ()
                n252 = property class="检测CTR"(reference=w287, "Value"=T4."Faild" ("值")) -> ()  [unwired: 1 in, 2 out]
                n253 = local write "STEP"("报表" ("F按钮名称（“取消”）")) -> ()
                n254 = call "设备状态.vi"("枚举"=w280, "工位"=w279, "Status_Write"=i16 400) -> ()  [unwired: 8 in, 1 out]
                n255 = call "合格状态.vi"("枚举"=w280, "工位"=w279, "Status_Write"=i16 2) -> ()  [unwired: 8 in, 1 out]
              }
              frame True {
                n256 = global read "Global.vi" "动态优化 2"() -> (w292)
                n257 = local read "判定结果"() -> (w288:bool[][])
                n258 = local write "STEP"("套输出轴") -> ()
                n259 = Build Array (concatenate)(w288, bool[][] [[TRUE, TRUE]] ("判定结果")) -> (w289:bool[][])
                n260 = local write "判定结果"(w289) -> ()
                n261 = property class="检测CTR"(reference=w292, "Value"=T4."Pass" ("值")) -> ()  [unwired: 1 in, 2 out]
              }
            }
          }
          frame "程序固化" {
            n262 = global read "Global.vi" "程序固化2引用句柄"() -> (w298)
            n263 = property class="检测CTR"(reference=w298) -> ("Value"=w297:variant)  [unwired: 1 in, 2 out]
            n264 = Variant To Data(type=检测CTR数据."Idle" ("Data"), Variant=w297) -> (data=w299:T2)  [unwired: 1 in, 1 out]
            n265 = Equal?(x=w299, y=检测CTR数据."Skip" ("Data")) -> (x = y?=w294:bool)
            n266 = case shown="假" w294 {
              frame False {
                n267 = stacked-sequence {
                  frame #0 {
                    n268 = global read "Global.vi" "程序固化引用句柄"() -> (w303:refnum<vi>)
                    n269 = property class="检测CTR"(reference=w303, "Value"=T4."Runing" ("值")) -> ()  [unwired: 1 in, 2 out]
                    n270 = call "设备状态.vi"("枚举"=enum16{"Read", "Write"}."Write", "工位"=enum16{"工位一", "工位二"}."工位二", "Status_Write"=i16 200) -> ()  [unwired: 8 in, 1 out]
                  }
                  frame #1 {
                    n271 = Wait (ms)(milliseconds to wait=u32 500 ("等待时间（毫秒）")) -> ()  [unwired: 1 out]
                  }
                  frame #2 {
                    n272 = local read "SENSOR"() -> (w309:T1)
                    n273 = call "FirmwareProgramming.vi"("SENSOR"=w309) -> ("Message"=w307:string, "Done?"=w308:bool)  [unwired: 8 in, 1 out]
                    n274 = case shown="真" w308 {
                      tunnel: w307 -> [w318 _]
                      tunnel: ["不合格" "报表"] -> w306
                      frame False {
                        n275 = global read "Global.vi" "程序固化2引用句柄"() -> (w320)
                        n276 = call "设备状态.vi"("枚举"=enum16{"Read", "Write"}."Write", "工位"=enum16{"工位一", "工位二"}."工位二", "Status_Write"=i16 400) -> ()  [unwired: 8 in, 1 out]
                        n277 = local read "判定结果"() -> (w313:bool[][])
                        n278 = Build Array (concatenate)(w313, bool[][] [[TRUE, FALSE]] ("判定结果")) -> (w315:bool[][])
                        n279 = Concatenate Strings("程序固化失败！\n可能的原因是：\n" ("字符串"), w318) -> (w317:string)
                        n280 = property class="检测CTR"(reference=w320, "Value"=T4."Faild" ("值")) -> ()  [unwired: 1 in, 2 out]
                        n281 = local write "判定结果"(w315) -> ()
                        n282 = One Button Dialog(message=w317) -> ()  [unwired: 1 in, 1 out]
                      }
                      frame True {
                        n283 = local read "判定结果"() -> (w325:bool[][])
                        n284 = global read "Global.vi" "程序固化2引用句柄"() -> (w329)
                        n285 = Build Array (concatenate)(w325, bool[][] [[TRUE, TRUE]] ("判定结果")) -> (w327:bool[][])
                        n286 = local write "判定结果"(w327) -> ()
                        n287 = property class="检测CTR"(reference=w329, "Value"=T4."Pass" ("值")) -> ()  [unwired: 1 in, 2 out]
                        n288 = call "设备状态.vi"("枚举"=enum16{"Read", "Write"}."Write", "工位"=enum16{"工位一", "工位二"}."工位二", "Status_Write"=i16 400) -> ()  [unwired: 8 in, 1 out]
                      }
                    }
                    n289 = local write "STEP"(w306) -> ()
                  }
                }
              }
              frame True {
                n290 = call "设备状态.vi"("枚举"=enum16{"Read", "Write"}."Write", "工位"=enum16{"工位一", "工位二"}."工位二", "Status_Write"=i16 400) -> ()  [unwired: 8 in, 1 out]
                n291 = local read "判定结果"() -> (w335:bool[][])
                n292 = local write "STEP"("报表" ("STEP")) -> ()
                n293 = Build Array (concatenate)(w335, bool[][] [[FALSE, FALSE]] ("判定结果")) -> (w337:bool[][])
                n294 = local write "判定结果"(w337) -> ()
              }
            }
          }
          frame "程序复检" {
            n295 = global read "Global.vi" "复检2引用句柄"() -> (w342)
            n296 = property class="检测CTR"(reference=w342) -> ("Value"=w343:variant)  [unwired: 1 in, 2 out]
            n297 = Variant To Data(type=检测CTR数据."Idle" ("Data"), Variant=w343) -> (data=w341:T2)  [unwired: 1 in, 1 out]
            n298 = Equal?(x=w341, y=检测CTR数据."Skip" ("Data")) -> (x = y?=w338:bool)
            n299 = case shown="真" w338 {
              frame False {
                n300 = stacked-sequence {
                  frame #0 {
                    n301 = call "浮动通知.vi"("通知内容"="程序复检" ("Status")) -> ()  [unwired: 11 in]
                    n302 = global read "Global.vi" "复检2引用句柄"() -> (w346)
                    n303 = local write "选项卡控件"(enum32{"工位二程序复检", "工位二动态复检"}."工位二程序复检" ("选项卡控件")) -> ()
                    n304 = property class="检测CTR"(reference=w346, "Value"=T4."Runing" ("值")) -> ()  [unwired: 1 in, 2 out]
                  }
                  frame #1 {
                    n305 = vi-ref "T1T2占空比2.vi"() -> (w349:refnum<vi>)
                    n306 = call "CallVI.vi"("VI引用"=w349, "状态"=T3."Hidden") -> ()  [unwired: 12 in, 2 out]
                    n307 = local write "STEP"("自动" ("STEP")) -> ()
                    n308 = call "设备状态.vi"("枚举"=enum16{"Read", "Write"}."Write", "工位"=enum16{"工位一", "工位二"}."工位二", "Status_Write"=i16 300) -> ()  [unwired: 8 in, 1 out]
                  }
                  frame #2 {
                    n309 = vi-ref "扭矩.vi"() -> (w355:refnum<vi>)
                    n310 = call "CallVI.vi"("VI引用"=w355, "状态"=T3."Hidden") -> ()  [unwired: 12 in, 2 out]
                  }
                }
              }
              frame True {
                n311 = local read "判定结果"() -> (w356:bool[][])
                n312 = local write "STEP"("程序固化" ("STEP")) -> ()
                n313 = Build Array (concatenate)(w356, bool[][] [[FALSE, FALSE]] ("判定结果")) -> (w358:bool[][])
                n314 = local write "判定结果"(w358) -> ()
              }
            }
          }
          frame "复检判定" {
            n315 = global read "Global.vi" "Result 2"() -> (w372)
            n316 = global read "Global.vi" "复检判定参数"() -> (w370:T7)
            n317 = local read "传感器复检"() -> (w371:cluster{dbl[], dbl[]}[])
            n318 = global read "Global.vi" "复检2引用句柄"() -> (w369)
            n319 = call "对中台复检判定.vi"("Result"=w372, "判定参数"=w370, "XY曲线"=w371) -> ("OK？"=w360:bool)  [unwired: 8 in]
            n320 = Select(t=T4."Pass" ("值"), s=w360, f=T4."Faild" ("值")) -> (s? t:f=w366:T4)
            n321 = Build Array(TRUE ("元素"), w360) -> (w362:bool[])
            n322 = local read "判定结果"() -> (w364:bool[][])
            n323 = property class="检测CTR"(reference=w369, "Value"=w366) -> ()  [unwired: 1 in, 2 out]
            n324 = Build Array(w362) -> (w361:bool[][])
            n325 = Build Array (concatenate)(w364, w361) -> (w365:bool[][])
            n326 = case shown="假" w360 {
              frame False {
                w385 = enum16{"Read", "Write"}."Write" ("枚举")
                n327 = call "设备状态.vi"("枚举"=w385, "工位"=enum16{"工位一", "工位二"}."工位二", "Status_Write"=i16 400) -> ()  [unwired: 8 in, 1 out]
                n328 = local write "STEP"("报表" ("STEP")) -> ()
                n329 = call "合格状态.vi"("枚举"=w385, "工位"=enum16{"工位一", "工位二"}."工位二", "Status_Write"=i16 2) -> ()  [unwired: 8 in, 1 out]
              }
              frame True {
                n330 = local write "STEP"("程序固化" ("STEP")) -> ()
              }
            }
            n331 = local write "判定结果"(w365) -> ()
            n332 = disable-structure shown="禁用" {
              frame Disabled {
                n333 = Two Button Dialog(message="复检失败\n请选择是否继续？" ("消息"), 1:"否" ("F按钮名称（“取消”）"), 2:"是" ("T按钮名称（“确定”）")) -> (T button?=w376:bool)
                n334 = case shown="假" w376 {
                  tunnel: ["报表" ("STEP") "程序固化" ("STEP")] -> w377
                  frame False {
                    n335 = call "设备状态.vi"("枚举"=enum16{"Read", "Write"}."Write", "工位"=enum16{"工位一", "工位二"}."工位一", "Status_Write"=i16 400) -> ()  [unwired: 8 in, 1 out]
                  }
                  frame True {
                  }
                }
                n336 = local write "STEP"(w377) -> ()
              }
              frame Enabled {
              }
            }
          }
          frame "自动" {
            n337 = call "设备状态.vi"("工位"=enum16{"工位一", "工位二"}."工位二") -> ("Status_Read"=w391:i16)  [unwired: 10 in]
            n338 = case shown="513" w391 {
              frame -128 {
                n339 = global write "Global.vi" "计时开始"(FALSE ("计时开始")) -> ()
                n340 = call "浮动通知.vi"("通知内容"="复位中……" ("Status")) -> ()  [unwired: 11 in]
              }
              frame 0, Default {
                n341 = disable-structure shown="禁用" {
                  frame Disabled {
                    n342 = global write "Global.vi" "计时开始"(FALSE ("计时开始")) -> ()
                  }
                  frame Enabled {
                  }
                }
              }
              frame 1 {
                n343 = call "浮动通知.vi"("通知内容"="请复位！" ("Status")) -> ()  [unwired: 11 in]
              }
              frame 5 {
                n344 = global write "Global.vi" "计时开始"(FALSE ("计时开始")) -> ()
                n345 = call "浮动通知.vi"("通知内容"="复位完成" ("Status")) -> ()  [unwired: 11 in]
              }
              frame 8 {
                n346 = call "浮动通知.vi"("通知内容"="程序停止！" ("Status")) -> ()  [unwired: 11 in]
              }
              frame 20 {
                n347 = local write "STEP"("扫码" ("STEP")) -> ()
              }
              frame 300 {
                n348 = call "设备状态.vi"("枚举"=enum16{"Read", "Write"}."Write", "工位"=enum16{"工位一", "工位二"}."工位二", "Status_Write"=i16 310) -> ()  [unwired: 8 in, 1 out]
              }
              frame 310 {
                n349 = call "传感器数据.vi"() -> ("传感器读数"=w404:T6)  [unwired: 11 in]
                n350 = global read "Global.vi" "扭矩"() -> (w416:cluster{"工位一":dbl, "工位二":dbl})
                n351 = Unbundle By Name(w404) -> ("工位二驱动伺服位移"=w405:sgl)
                n352 = global read "Global.vi" "保护角度"() -> (w409:dbl)
                n353 = Unbundle By Name(w416) -> ("工位二"=w412:dbl)
                n354 = local read "初始角度"() -> (w406:dbl)
                n355 = Subtract(x=w405, y=w406) -> (x-y=w407:dbl)
                n356 = Subtract(x=w412, y=-0.05) -> (x-y=w413:dbl)
                n357 = Absolute Value(x=w407) -> (abs(x)=w408:dbl)
                n358 = Less Or Equal?(x=w413, y=-6.0) -> (x <= y?=w411:bool)
                n359 = Greater Or Equal?(x=w408, y=w409) -> (x >= y?=w403:bool)
                n360 = Compound Arithmetic op=OR ("复合运算")(w411, w403) -> (w410:bool)
                n361 = case shown="假" w410 {
                  tunnel: w412 -> [w417 _]
                  tunnel: w403 -> [_ w439]
                  frame False {
                    n362 = feedback #1() -> (w434:dbl)  [unwired: 1 in]
                    n363 = feedback-in #1(w417) -> ()
                    n364 = feedback #2() -> (w425:dbl)  [unwired: 1 in]
                    n365 = Equal?(x=w417, y=w434) -> (x = y?=w432:bool)
                    n366 = feedback #3() -> (w433:dbl)  [unwired: 1 in]
                    n367 = feedback-in #3(w434) -> ()
                    n368 = feedback #4() -> (w424:dbl)  [unwired: 1 in]
                    n369 = feedback-in #4(w425) -> ()
                    n370 = Equal?(x=w417, y=w425) -> (x = y?=w422:bool)
                    n371 = feedback #5() -> (w423:dbl)  [unwired: 1 in]
                    n372 = feedback-in #5(w424) -> ()
                    n373 = Equal?(x=w417, y=w433) -> (x = y?=w431:bool)
                    n374 = Equal?(x=w417, y=w424) -> (x = y?=w421:bool)
                    n375 = feedback #6() -> (w428:dbl)  [unwired: 1 in]
                    n376 = feedback-in #6(w433) -> ()
                    n377 = feedback #7() -> (w418:dbl)  [unwired: 1 in]
                    n378 = feedback-in #7(w423) -> ()
                    n379 = Equal?(x=w417, y=w428) -> (x = y?=w430:bool)
                    n380 = feedback #8() -> (w426:dbl)  [unwired: 1 in]
                    n381 = feedback-in #2(w426) -> ()
                    n382 = feedback-in #8(w428) -> ()
                    n383 = Equal?(x=w417, y=w423) -> (x = y?=w420:bool)
                    n384 = Equal?(x=w417, y=w426) -> (x = y?=w427:bool)
                    n385 = Equal?(x=w417, y=w418) -> (x = y?=w419:bool)
                    n386 = Compound Arithmetic op=AND(w432, w431, w430, w427, w422, w421, w420, w419) -> (w429:bool)
                    n387 = case shown="真" w429 {
                      frame False {
                      }
                      frame True {
                        n388 = call "设备状态.vi"("枚举"=enum16{"Read", "Write"}."Write", "工位"=enum16{"工位一", "工位二"}."工位二", "Status_Write"=i16 316) -> ()  [unwired: 8 in, 1 out]
                        n389 = One Button Dialog(message="扭矩采集异常！\n请重启应用程序！" ("消息")) -> ()  [unwired: 1 in, 1 out]
                      }
                    }
                  }
                  frame True {
                    n390 = case shown="真" w439 {
                      frame False {
                        n391 = call "设备状态.vi"("枚举"=enum16{"Read", "Write"}."Write", "工位"=enum16{"工位一", "工位二"}."工位一", "Status_Write"=i16 311) -> ()  [unwired: 8 in, 1 out]
                      }
                      frame True {
                        n392 = call "设备状态.vi"("枚举"=enum16{"Read", "Write"}."Write", "工位"=enum16{"工位一", "工位二"}."工位一", "Status_Write"=i16 316) -> ()  [unwired: 8 in, 1 out]
                        n393 = One Button Dialog(message="扭矩采集异常！\n请重启应用程序！" ("消息")) -> ()  [unwired: 1 in, 1 out]
                      }
                    }
                  }
                }
              }
              frame 311 {
                n394 = global read "Global.vi" "扭矩"() -> (w451:cluster{"工位一":dbl, "工位二":dbl})
                n395 = Unbundle By Name(w451) -> ("工位二"=w450:dbl)
                n396 = Subtract(x=w450, y=0.3) -> (x-y=w449:dbl)
                n397 = Greater Or Equal To 0?(x=w449) -> (x >= 0?=w448:bool)
                n398 = case shown="假" w448 {
                  frame False {
                  }
                  frame True {
                    n399 = call "设备状态.vi"("枚举"=enum16{"Read", "Write"}."Write", "工位"=enum16{"工位一", "工位二"}."工位二", "Status_Write"=i16 312) -> ()  [unwired: 8 in, 1 out]
                  }
                }
              }
              frame 312 {
                n400 = global read "Global.vi" "工位一扭矩偏移"() -> (w464:cluster{"正向":dbl, "逆向":dbl})
                n401 = call "传感器数据.vi"() -> ("传感器读数"=w456:T6)  [unwired: 11 in]
                n402 = Unbundle By Name(w456) -> ("工位二驱动伺服位移"=w457:sgl)
                n403 = global read "Global.vi" "扭矩"() -> (w470:cluster{"工位一":dbl, "工位二":dbl})
                n404 = global read "Global.vi" "保护角度"() -> (w461:dbl)
                n405 = local read "初始角度"() -> (w458:dbl)
                n406 = global read "Global.vi" "复检参数"() -> (w469:T8)
                n407 = Unbundle By Name(w470) -> ("工位二"=w466:dbl)
                n408 = Unbundle By Name(w464) -> ()  [unwired: 1 out]
                n409 = Subtract(x=w457, y=w458) -> (x-y=w459:dbl)
                n410 = Unbundle By Name(w469) -> ("换向扭矩"=w468:dbl)
                n411 = Subtract(x=w466, y=0.3) -> (x-y=w465:dbl)
                n412 = Absolute Value(x=w459) -> (abs(x)=w460:dbl)
                n413 = Greater Or Equal?(x=w460, y=w461) -> (x >= y?=w455:bool)
                n414 = Greater?(x=w465, y=w468) -> (0:w467:bool)
                n415 = Compound Arithmetic op=OR ("复合运算")(w467, w455) -> (w462:bool)
                n416 = case shown="真" w462 {
                  tunnel: w465 -> [w473 _]
                  tunnel: w455 -> [_ w522]
                  frame False {
                    n417 = local read "传感器复检"() -> (w474:cluster{dbl[], dbl[]}[])
                    n418 = local read "初始化"() -> (w472:bool[])
                    n419 = for {
                      tunnel: w474 -> [w480] mode=indexing
                      tunnel: [w479] -> w475 mode=indexing
                      tunnel: w473 -> [w478]
                      tunnel: w472 -> [w477] mode=indexing
                      tunnel: [w476] -> w471 mode=indexing
                      i -> [w481]
                      n420 = case shown="2" w481 {
                        tunnel: w480 -> [w483 w492 w504 w518]
                        tunnel: [w483 w490 w502 w514] -> w479
                        tunnel: w478 -> [_ w489 w500 w512]
                        tunnel: w477 -> [w482 w484 w498 w508]
                        tunnel: [w482 FALSE ("布尔") FALSE ("布尔") FALSE ("布尔")] -> w476
                        frame Default {
                        }
                        frame 0 {
                          n421 = call <vilib>:"Median Filter PtByPt.vi"("initialize"=w484, "x"=w489) -> ("Filtered x"=w488:dbl)  [unwired: 2 in, 1 out]
                          n422 = Unbundle(w492) -> (w495:dbl[], w491:dbl[])
                          n423 = global read "Global.vi" "工位一T1"() -> (w487:dbl)
                          n424 = Build Array (concatenate)(w495, w488) -> (w494:dbl[])
                          n425 = call <vilib>:"Median Filter PtByPt.vi"("initialize"=w484, "x"=w487) -> ("Filtered x"=w486:dbl)  [unwired: 2 in, 1 out]
                          n426 = Build Array (concatenate)(w491, w486) -> (w493:dbl[])
                          n427 = Bundle(w494, w493) -> (w490:cluster{dbl[], dbl[]})  [unwired: 1 in]
                        }
                        frame 1 {
                          n428 = call <vilib>:"Median Filter PtByPt.vi"("initialize"=w498, "x"=w500) -> ("Filtered x"=w499:dbl)  [unwired: 2 in, 1 out]
                          n429 = Unbundle(w504) -> (w507:dbl[], w503:dbl[])
                          n430 = global read "Global.vi" "工位一T2"() -> (w497:dbl)
                          n431 = Build Array (concatenate)(w507, w499) -> (w506:dbl[])
                          n432 = call <vilib>:"Median Filter PtByPt.vi"("initialize"=w498, "x"=w497) -> ("Filtered x"=w496:dbl)  [unwired: 2 in, 1 out]
                          n433 = Build Array (concatenate)(w503, w496) -> (w505:dbl[])
                          n434 = Bundle(w506, w505) -> (w502:cluster{dbl[], dbl[]})  [unwired: 1 in]
                        }
                        frame 2 {
                          n435 = call <vilib>:"Median Filter PtByPt.vi"("initialize"=w508, "x"=w512) -> ("Filtered x"=w511:dbl)  [unwired: 2 in, 1 out]
                          n436 = Unbundle(w518) -> (w521:dbl[], w517:dbl[])
                          n437 = global read "Global.vi" "工位一T1"() -> (w516:dbl)
                          n438 = global read "Global.vi" "工位一T2"() -> (w515:dbl)
                          n439 = Build Array (concatenate)(w521, w511) -> (w520:dbl[])
                          n440 = Add(x=w516, y=w515) -> (x+y=w510:dbl)
                          n441 = call <vilib>:"Median Filter PtByPt.vi"("initialize"=w508, "x"=w510) -> ("Filtered x"=w509:dbl)  [unwired: 2 in, 1 out]
                          n442 = Build Array (concatenate)(w517, w509) -> (w519:dbl[])
                          n443 = Bundle(w520, w519) -> (w514:cluster{dbl[], dbl[]})  [unwired: 1 in]
                        }
                      }
                    }
                    n444 = local write "初始化"(w471) -> ()
                    n445 = local write "传感器复检"(w475) -> ()
                  }
                  frame True {
                    n446 = case shown="真" w522 {
                      frame False {
                        n447 = call "设备状态.vi"("枚举"=enum16{"Read", "Write"}."Write", "工位"=enum16{"工位一", "工位二"}."工位一", "Status_Write"=i16 313) -> ()  [unwired: 8 in, 1 out]
                      }
                      frame True {
                        n448 = call "设备状态.vi"("枚举"=enum16{"Read", "Write"}."Write", "工位"=enum16{"工位一", "工位二"}."工位二", "Status_Write"=i16 316) -> ()  [unwired: 8 in, 1 out]
                        n449 = One Button Dialog(message="扭矩采集异常！\n请重启应用程序！" ("消息")) -> ()  [unwired: 1 in, 1 out]
                      }
                    }
                  }
                }
              }
              frame 313 {
                n450 = global read "Global.vi" "工位一扭矩偏移"() -> (w536:cluster{"正向":dbl, "逆向":dbl})
                n451 = global read "Global.vi" "扭矩"() -> (w538:cluster{"工位一":dbl, "工位二":dbl})
                n452 = global read "Global.vi" "复检参数"() -> (w533:T8)
                n453 = Unbundle By Name(w538) -> ("工位二"=w535:dbl)
                n454 = Unbundle By Name(w536) -> ()  [unwired: 1 out]
                n455 = Unbundle By Name(w533) -> ("换向扭矩"=w531:dbl)
                n456 = Subtract(x=w535, y=-0.05) -> (x-y=w532:dbl)
                n457 = Less Or Equal To 0?(x=w532) -> (x <= 0?=w537:bool)
                n458 = Less?(x=w532, y=w531) -> (x < y?=w530:bool)
                n459 = case shown="真" w537 {
                  tunnel: w532 -> [w540 _]
                  tunnel: w530 -> [w539 _]
                  frame False {
                    n460 = case shown="假" w539 {
                      tunnel: w540 -> [_ w543]
                      frame False {
                      }
                      frame True {
                        n461 = local read "传感器复检"() -> (w544:cluster{dbl[], dbl[]}[])
                        n462 = local read "初始化"() -> (w542:bool[])
                        n463 = for {
                          tunnel: w544 -> [w550] mode=indexing
                          tunnel: [w549] -> w545 mode=indexing
                          tunnel: w543 -> [w548]
                          tunnel: w542 -> [w547] mode=indexing
                          tunnel: [w546] -> w541 mode=indexing
                          i -> [w551]
                          n464 = case shown="默认" w551 {
                            tunnel: w550 -> [w553 w562 w574 w588]
                            tunnel: [w553 w560 w572 w584] -> w549
                            tunnel: w548 -> [_ w558 w570 w582]
                            tunnel: w547 -> [w552 w554 w571 w583]
                            tunnel: [w552 FALSE ("布尔") FALSE ("布尔") FALSE ("布尔")] -> w546
                            frame Default {
                            }
                            frame 3 {
                              n465 = call <vilib>:"Median Filter PtByPt.vi"("initialize"=w554, "x"=w558) -> ("Filtered x"=w557:dbl)  [unwired: 2 in, 1 out]
                              n466 = Unbundle(w562) -> (w565:dbl[], w561:dbl[])
                              n467 = global read "Global.vi" "工位一T1"() -> (w556:dbl)
                              n468 = Build Array (concatenate)(w565, w557) -> (w564:dbl[])
                              n469 = call <vilib>:"Median Filter PtByPt.vi"("initialize"=w554, "x"=w556) -> ("Filtered x"=w555:dbl)  [unwired: 2 in, 1 out]
                              n470 = Build Array (concatenate)(w561, w555) -> (w563:dbl[])
                              n471 = Bundle(w564, w563) -> (w560:cluster{dbl[], dbl[]})  [unwired: 1 in]
                            }
                            frame 4 {
                              n472 = call <vilib>:"Median Filter PtByPt.vi"("initialize"=w571, "x"=w570) -> ("Filtered x"=w569:dbl)  [unwired: 2 in, 1 out]
                              n473 = Unbundle(w574) -> (w577:dbl[], w573:dbl[])
                              n474 = global read "Global.vi" "工位一T2"() -> (w568:dbl)
                              n475 = Build Array (concatenate)(w577, w569) -> (w576:dbl[])
                              n476 = call <vilib>:"Median Filter PtByPt.vi"("initialize"=w571, "x"=w568) -> ("Filtered x"=w567:dbl)  [unwired: 2 in, 1 out]
                              n477 = Build Array (concatenate)(w573, w567) -> (w575:dbl[])
                              n478 = Bundle(w576, w575) -> (w572:cluster{dbl[], dbl[]})  [unwired: 1 in]
                            }
                            frame 5 {
                              n479 = call <vilib>:"Median Filter PtByPt.vi"("initialize"=w583, "x"=w582) -> ("Filtered x"=w581:dbl)  [unwired: 2 in, 1 out]
                              n480 = Unbundle(w588) -> (w591:dbl[], w587:dbl[])
                              n481 = global read "Global.vi" "工位一T1"() -> (w586:dbl)
                              n482 = global read "Global.vi" "工位一T2"() -> (w585:dbl)
                              n483 = Build Array (concatenate)(w591, w581) -> (w590:dbl[])
                              n484 = Add(x=w586, y=w585) -> (x+y=w580:dbl)
                              n485 = call <vilib>:"Median Filter PtByPt.vi"("initialize"=w583, "x"=w580) -> ("Filtered x"=w579:dbl)  [unwired: 2 in, 1 out]
                              n486 = Build Array (concatenate)(w587, w579) -> (w589:dbl[])
                              n487 = Bundle(w590, w589) -> (w584:cluster{dbl[], dbl[]})  [unwired: 1 in]
                            }
                          }
                        }
                        n488 = local write "初始化"(w541) -> ()
                        n489 = local write "传感器复检"(w545) -> ()
                      }
                    }
                  }
                  frame True {
                    n490 = call "设备状态.vi"("枚举"=enum16{"Read", "Write"}."Write", "工位"=enum16{"工位一", "工位二"}."工位二", "Status_Write"=i16 314) -> ()  [unwired: 8 in, 1 out]
                  }
                }
              }
              frame 314 {
                n491 = global read "Global.vi" "工位一扭矩偏移"() -> (w606:cluster{"正向":dbl, "逆向":dbl})
                n492 = call "传感器数据.vi"() -> ("传感器读数"=w597:T6)  [unwired: 11 in]
                n493 = global read "Global.vi" "复检参数"() -> (w609:T8)
                n494 = Unbundle By Name(w597) -> ("工位二驱动伺服位移"=w598:sgl)
                n495 = global read "Global.vi" "扭矩"() -> (w610:cluster{"工位一":dbl, "工位二":dbl})
                n496 = global read "Global.vi" "保护角度"() -> (w602:dbl)
                n497 = Unbundle By Name(w609) -> ("换向扭矩"=w608:dbl)
                n498 = local read "初始角度"() -> (w599:dbl)
                n499 = Unbundle By Name(w610) -> ("工位二"=w605:dbl)
                n500 = Unbundle By Name(w606) -> ()  [unwired: 1 out]
                n501 = Subtract(x=w598, y=w599) -> (x-y=w600:dbl)
                n502 = Negate(x=w608) -> (-x=w611:dbl)
                n503 = Subtract(x=w605, y=-0.05) -> (x-y=w603:dbl)
                n504 = Absolute Value(x=w600) -> (abs(x)=w601:dbl)
                n505 = Less Or Equal?(x=w603, y=w611) -> (x <= y?=w607:bool)
                n506 = Greater Or Equal?(x=w601, y=w602) -> (x >= y?=w595:bool)
                n507 = Compound Arithmetic op=OR ("复合运算")(w607, w595) -> (w596:bool)
                n508 = case shown="假" w596 {
                  tunnel: w603 -> [w614 _]
                  tunnel: w603 -> [w612 _]
                  tunnel: w595 -> [_ w666]
                  frame False {
                    n509 = Less Or Equal To 0?(x=w612) -> (x <= 0?=w613:bool)
                    n510 = case shown="真" w613 {
                      tunnel: w614 -> [_ w617]
                      frame False {
                      }
                      frame True {
                        n511 = local read "传感器复检"() -> (w618:cluster{dbl[], dbl[]}[])
                        n512 = local read "初始化"() -> (w616:bool[])
                        n513 = for {
                          tunnel: w618 -> [w624] mode=indexing
                          tunnel: [w623] -> w619 mode=indexing
                          tunnel: w617 -> [w622]
                          tunnel: w616 -> [w621] mode=indexing
                          tunnel: [w620] -> w615 mode=indexing
                          i -> [w625]
                          n514 = case shown="默认" w625 {
                            tunnel: w624 -> [w627 w636 w648 w662]
                            tunnel: [w627 w634 w646 w658] -> w623
                            tunnel: w622 -> [_ w633 w645 w657]
                            tunnel: w621 -> [w626 w629 w641 w653]
                            tunnel: [w626 FALSE ("布尔") FALSE ("布尔") FALSE ("布尔")] -> w620
                            frame Default {
                            }
                            frame 6 {
                              n515 = call <vilib>:"Median Filter PtByPt.vi"("initialize"=w629, "x"=w633) -> ("Filtered x"=w632:dbl)  [unwired: 2 in, 1 out]
                              n516 = Unbundle(w636) -> (w639:dbl[], w635:dbl[])
                              n517 = global read "Global.vi" "工位一T1"() -> (w631:dbl)
                              n518 = Build Array (concatenate)(w639, w632) -> (w638:dbl[])
                              n519 = call <vilib>:"Median Filter PtByPt.vi"("initialize"=w629, "x"=w631) -> ("Filtered x"=w630:dbl)  [unwired: 2 in, 1 out]
                              n520 = Build Array (concatenate)(w635, w630) -> (w637:dbl[])
                              n521 = Bundle(w638, w637) -> (w634:cluster{dbl[], dbl[]})  [unwired: 1 in]
                            }
                            frame 7 {
                              n522 = call <vilib>:"Median Filter PtByPt.vi"("initialize"=w641, "x"=w645) -> ("Filtered x"=w644:dbl)  [unwired: 2 in, 1 out]
                              n523 = Unbundle(w648) -> (w651:dbl[], w647:dbl[])
                              n524 = global read "Global.vi" "工位一T2"() -> (w643:dbl)
                              n525 = Build Array (concatenate)(w651, w644) -> (w650:dbl[])
                              n526 = call <vilib>:"Median Filter PtByPt.vi"("initialize"=w641, "x"=w643) -> ("Filtered x"=w642:dbl)  [unwired: 2 in, 1 out]
                              n527 = Build Array (concatenate)(w647, w642) -> (w649:dbl[])
                              n528 = Bundle(w650, w649) -> (w646:cluster{dbl[], dbl[]})  [unwired: 1 in]
                            }
                            frame 8 {
                              n529 = call <vilib>:"Median Filter PtByPt.vi"("initialize"=w653, "x"=w657) -> ("Filtered x"=w656:dbl)  [unwired: 2 in, 1 out]
                              n530 = Unbundle(w662) -> (w665:dbl[], w661:dbl[])
                              n531 = global read "Global.vi" "工位一T1"() -> (w660:dbl)
                              n532 = global read "Global.vi" "工位一T2"() -> (w659:dbl)
                              n533 = Build Array (concatenate)(w665, w656) -> (w664:dbl[])
                              n534 = Add(x=w660, y=w659) -> (x+y=w655:dbl)
                              n535 = call <vilib>:"Median Filter PtByPt.vi"("initialize"=w653, "x"=w655) -> ("Filtered x"=w654:dbl)  [unwired: 2 in, 1 out]
                              n536 = Build Array (concatenate)(w661, w654) -> (w663:dbl[])
                              n537 = Bundle(w664, w663) -> (w658:cluster{dbl[], dbl[]})  [unwired: 1 in]
                            }
                          }
                        }
                        n538 = local write "初始化"(w615) -> ()
                        n539 = local write "传感器复检"(w619) -> ()
                      }
                    }
                  }
                  frame True {
                    n540 = case shown="假" w666 {
                      frame False {
                        n541 = call "设备状态.vi"("枚举"=enum16{"Read", "Write"}."Write", "工位"=enum16{"工位一", "工位二"}."工位二", "Status_Write"=i16 315) -> ()  [unwired: 8 in, 1 out]
                      }
                      frame True {
                        n542 = call "设备状态.vi"("枚举"=enum16{"Read", "Write"}."Write", "工位"=enum16{"工位一", "工位二"}."工位二", "Status_Write"=i16 316) -> ()  [unwired: 8 in, 1 out]
                        n543 = One Button Dialog(message="扭矩采集异常！\n请重启应用程序！" ("消息")) -> ()  [unwired: 1 in, 1 out]
                      }
                    }
                  }
                }
              }
              frame 315 {
                n544 = global read "Global.vi" "工位一扭矩偏移"() -> (w680:cluster{"正向":dbl, "逆向":dbl})
                n545 = global read "Global.vi" "复检参数"() -> (w677:T8)
                n546 = global read "Global.vi" "扭矩"() -> (w683:cluster{"工位一":dbl, "工位二":dbl})
                n547 = Unbundle By Name(w677) -> ("换向扭矩"=w676:dbl)
                n548 = Unbundle By Name(w683) -> ("工位二"=w679:dbl)
                n549 = Unbundle By Name(w680) -> ()  [unwired: 1 out]
                n550 = Negate(x=w676) -> (-x=w675:dbl)
                n551 = Subtract(x=w679, y=0.3) -> (x-y=w674:dbl)
                n552 = Greater?(x=w674, y=0.0) -> (0:w682:bool)
                n553 = case shown="真" w682 {
                  tunnel: w674 -> [w687 _]
                  tunnel: w675 -> [w685 _]
                  tunnel: w674 -> [w684 _]
                  frame False {
                    n554 = Greater Or Equal?(x=w684, y=w685) -> (x >= y?=w686:bool)
                    n555 = case shown="假" w686 {
                      tunnel: w687 -> [_ w690]
                      frame False {
                      }
                      frame True {
                        n556 = local read "传感器复检"() -> (w691:cluster{dbl[], dbl[]}[])
                        n557 = local read "初始化"() -> (w689:bool[])
                        n558 = for {
                          tunnel: w691 -> [w697] mode=indexing
                          tunnel: [w696] -> w692 mode=indexing
                          tunnel: w690 -> [w695]
                          tunnel: w689 -> [w694] mode=indexing
                          tunnel: [w693] -> w688 mode=indexing
                          i -> [w698]
                          n559 = case shown="11" w698 {
                            tunnel: w697 -> [w700 w709 w721 w735]
                            tunnel: [w700 w707 w719 w731] -> w696
                            tunnel: w695 -> [_ w705 w717 w729]
                            tunnel: w694 -> [w699 w706 w713 w730]
                            tunnel: [w699 FALSE ("布尔") FALSE ("布尔") FALSE ("布尔")] -> w693
                            frame Default {
                            }
                            frame 9 {
                              n560 = call <vilib>:"Median Filter PtByPt.vi"("initialize"=w706, "x"=w705) -> ("Filtered x"=w704:dbl)  [unwired: 2 in, 1 out]
                              n561 = Unbundle(w709) -> (w712:dbl[], w708:dbl[])
                              n562 = global read "Global.vi" "工位二T1"() -> (w703:dbl)
                              n563 = Build Array (concatenate)(w712, w704) -> (w711:dbl[])
                              n564 = call <vilib>:"Median Filter PtByPt.vi"("initialize"=w706, "x"=w703) -> ("Filtered x"=w702:dbl)  [unwired: 2 in, 1 out]
                              n565 = Build Array (concatenate)(w708, w702) -> (w710:dbl[])
                              n566 = Bundle(w711, w710) -> (w707:cluster{dbl[], dbl[]})  [unwired: 1 in]
                            }
                            frame 10 {
                              n567 = call <vilib>:"Median Filter PtByPt.vi"("initialize"=w713, "x"=w717) -> ("Filtered x"=w716:dbl)  [unwired: 2 in, 1 out]
                              n568 = Unbundle(w721) -> (w724:dbl[], w720:dbl[])
                              n569 = global read "Global.vi" "工位二T2"() -> (w715:dbl)
                              n570 = Build Array (concatenate)(w724, w716) -> (w723:dbl[])
                              n571 = call <vilib>:"Median Filter PtByPt.vi"("initialize"=w713, "x"=w715) -> ("Filtered x"=w714:dbl)  [unwired: 2 in, 1 out]
                              n572 = Build Array (concatenate)(w720, w714) -> (w722:dbl[])
                              n573 = Bundle(w723, w722) -> (w719:cluster{dbl[], dbl[]})  [unwired: 1 in]
                            }
                            frame 11 {
                              n574 = call <vilib>:"Median Filter PtByPt.vi"("initialize"=w730, "x"=w729) -> ("Filtered x"=w728:dbl)  [unwired: 2 in, 1 out]
                              n575 = Unbundle(w735) -> (w738:dbl[], w734:dbl[])
                              n576 = global read "Global.vi" "工位二T1"() -> (w733:dbl)
                              n577 = global read "Global.vi" "工位二T2"() -> (w732:dbl)
                              n578 = Build Array (concatenate)(w738, w728) -> (w737:dbl[])
                              n579 = Add(x=w733, y=w732) -> (x+y=w727:dbl)
                              n580 = call <vilib>:"Median Filter PtByPt.vi"("initialize"=w730, "x"=w727) -> ("Filtered x"=w726:dbl)  [unwired: 2 in, 1 out]
                              n581 = Build Array (concatenate)(w734, w726) -> (w736:dbl[])
                              n582 = Bundle(w737, w736) -> (w731:cluster{dbl[], dbl[]})  [unwired: 1 in]
                            }
                          }
                        }
                        n583 = local write "初始化"(w688) -> ()
                        n584 = local write "传感器复检"(w692) -> ()
                      }
                    }
                  }
                  frame True {
                    n585 = call "设备状态.vi"("枚举"=enum16{"Read", "Write"}."Write", "工位"=enum16{"工位一", "工位二"}."工位二", "Status_Write"=i16 316) -> ()  [unwired: 8 in, 1 out]
                  }
                }
              }
              frame 316 {
                n586 = global write "Global.vi" "工位二占空比采集"(FALSE ("工位二占空比采集")) -> ()
                n587 = local write "STEP"("复检判定" ("STEP")) -> ()
              }
              frame 401 {
                n588 = call "设备状态.vi"("枚举"=enum16{"Read", "Write"}."Write", "工位"=enum16{"工位一", "工位二"}."工位二", "Status_Write"=i16 10) -> ()  [unwired: 8 in, 1 out]
              }
              frame 500 {
                n589 = global read "Global.vi" "动态优化完成"() -> (w748:bool)
                n590 = case shown="真" w748 {
                  frame False {
                    n591 = call "传感器数据.vi"() -> ("传感器读数"=w761:T6)  [unwired: 11 in]
                    n592 = Unbundle By Name(w761) -> ("工位二驱动伺服位移"=w763:sgl)
                    n593 = local read "动优化态前"() -> (w762:cluster{dbl[], dbl[]}[])
                    n594 = local read "初始化 3"() -> (w760:bool[])
                    n595 = for {
                      tunnel: [w770] -> w758 mode=indexing
                      tunnel: w763 -> [w769]
                      tunnel: w762 -> [w768] mode=indexing
                      tunnel: w760 -> [w766] mode=indexing
                      tunnel: [w765] -> w759 mode=indexing
                      i -> [w767]
                      n596 = case shown="3" w767 {
                        tunnel: [w772 w780 w790 w803 w816] -> w770
                        tunnel: w769 -> [_ w773 w783 w795 w808]
                        tunnel: w768 -> [w772 w778 w787 w800 w813]
                        tunnel: w766 -> [w771 w776 w785 w798 w811]
                        tunnel: [w771 FALSE ("布尔") FALSE ("布尔") FALSE ("布尔") FALSE ("布尔")] -> w765
                        tunnel: 4 ("rank") -> [_ _ _ w793 w806]
                        frame Default {
                        }
                        frame 0 {
                          n597 = call <vilib>:"Median Filter PtByPt.vi"("initialize"=w776) -> ()  [unwired: 3 in, 2 out]
                          n598 = Unbundle(w778) -> (w777:dbl[], w779:dbl[])
                          n599 = global read "Global.vi" "工位二T1"() -> (w774:dbl)
                          n600 = Build Array (concatenate)(w777, w773) -> (w782:dbl[])
                          n601 = call <vilib>:"Median Filter PtByPt.vi"("initialize"=w776) -> ()  [unwired: 3 in, 2 out]
                          n602 = Build Array (concatenate)(w779, w774) -> (w781:dbl[])
                          n603 = Bundle(w782, w781) -> (w780:cluster{dbl[], dbl[]})  [unwired: 1 in]
                        }
                        frame 1 {
                          n604 = Unbundle(w787) -> (w789:dbl[], w788:dbl[])
                          n605 = global read "Global.vi" "工位二T2"() -> (w784:dbl)
                          n606 = call <vilib>:"Median Filter PtByPt.vi"("initialize"=w785) -> ()  [unwired: 3 in, 2 out]
                          n607 = Build Array (concatenate)(w789, w783) -> (w792:dbl[])
                          n608 = Build Array (concatenate)(w788, w784) -> (w791:dbl[])
                          n609 = call <vilib>:"Median Filter PtByPt.vi"("initialize"=w785) -> ()  [unwired: 3 in, 2 out]
                          n610 = Bundle(w792, w791) -> (w790:cluster{dbl[], dbl[]})  [unwired: 1 in]
                        }
                        frame 2 {
                          n611 = global read "Global.vi" "工位一P"() -> (w797:dbl)
                          n612 = Unbundle(w800) -> (w802:dbl[], w801:dbl[])
                          n613 = call <vilib>:"Median Filter PtByPt.vi"("initialize"=w798, "rank"=w793, "x"=w795) -> ("Filtered x"=w794:dbl)  [unwired: 1 in, 1 out]
                          n614 = Build Array (concatenate)(w802, w794) -> (w805:dbl[])
                          n615 = call <vilib>:"Median Filter PtByPt.vi"("initialize"=w798, "rank"=w793, "x"=w797) -> ("Filtered x"=w796:dbl)  [unwired: 1 in, 1 out]
                          n616 = Build Array (concatenate)(w801, w796) -> (w804:dbl[])
                          n617 = Bundle(w805, w804) -> (w803:cluster{dbl[], dbl[]})  [unwired: 1 in]
                        }
                        frame 3 {
                          n618 = Unbundle(w813) -> (w815:dbl[], w814:dbl[])
                          n619 = call <vilib>:"Median Filter PtByPt.vi"("initialize"=w811, "rank"=w806, "x"=w808) -> ("Filtered x"=w807:dbl)  [unwired: 1 in, 1 out]
                          n620 = global read "Global.vi" "工位一S"() -> (w809:dbl)
                          n621 = Build Array (concatenate)(w815, w807) -> (w818:dbl[])
                          n622 = call <vilib>:"Median Filter PtByPt.vi"("initialize"=w811, "rank"=w806, "x"=w809) -> ("Filtered x"=w810:dbl)  [unwired: 1 in, 1 out]
                          n623 = Build Array (concatenate)(w814, w810) -> (w817:dbl[])
                          n624 = Bundle(w818, w817) -> (w816:cluster{dbl[], dbl[]})  [unwired: 1 in]
                        }
                      }
                    }
                    n625 = local write "初始化 3"(w759) -> ()
                    n626 = local write "动优化态前"(w758) -> ()
                    n627 = call "VRES值.vi"("XY"=w758, "索引1"=2, "索引2"=3) -> ("XY图 2"=w757:cluster{dbl[], dbl[]}[])  [unwired: 16 in]
                    n628 = Index Array(array=w757, index=8 ("索引")) -> (element=→"VRES_cW":cluster{dbl[], dbl[]})
                  }
                  frame True {
                    n629 = call "传感器数据.vi"() -> ("传感器读数"=w822:T6)  [unwired: 11 in]
                    n630 = Unbundle By Name(w822) -> ("工位二驱动伺服位移"=w824:sgl)
                    n631 = local read "动优化态"() -> (w823:cluster{dbl[], dbl[]}[])
                    n632 = local read "初始化 2"() -> (w821:bool[])
                    n633 = for {
                      tunnel: [w831] -> w819 mode=indexing
                      tunnel: w824 -> [w830]
                      tunnel: w823 -> [w829] mode=indexing
                      tunnel: w821 -> [w827] mode=indexing
                      tunnel: [w826] -> w820 mode=indexing
                      i -> [w828]
                      n634 = case shown="2" w828 {
                        tunnel: [w833 w841 w851 w866] -> w831
                        tunnel: w830 -> [_ w834 w844 w859]
                        tunnel: w829 -> [w833 w839 w848 w863]
                        tunnel: w827 -> [w832 w837 w846 w861]
                        tunnel: [w832 FALSE ("布尔") FALSE ("布尔") FALSE ("布尔")] -> w826
                        tunnel: 4 ("rank") -> [_ _ _ w857]
                        frame Default {
                        }
                        frame 0 {
                          n635 = call <vilib>:"Median Filter PtByPt.vi"("initialize"=w837) -> ()  [unwired: 3 in, 2 out]
                          n636 = Unbundle(w839) -> (w838:dbl[], w840:dbl[])
                          n637 = global read "Global.vi" "工位二T1"() -> (w835:dbl)
                          n638 = Build Array (concatenate)(w838, w834) -> (w843:dbl[])
                          n639 = call <vilib>:"Median Filter PtByPt.vi"("initialize"=w837) -> ()  [unwired: 3 in, 2 out]
                          n640 = Build Array (concatenate)(w840, w835) -> (w842:dbl[])
                          n641 = Bundle(w843, w842) -> (w841:cluster{dbl[], dbl[]})  [unwired: 1 in]
                        }
                        frame 1 {
                          n642 = Unbundle(w848) -> (w850:dbl[], w849:dbl[])
                          n643 = global read "Global.vi" "工位二T2"() -> (w845:dbl)
                          n644 = call <vilib>:"Median Filter PtByPt.vi"("initialize"=w846) -> ()  [unwired: 3 in, 2 out]
                          n645 = Build Array (concatenate)(w850, w844) -> (w853:dbl[])
                          n646 = Build Array (concatenate)(w849, w845) -> (w852:dbl[])
                          n647 = call <vilib>:"Median Filter PtByPt.vi"("initialize"=w846) -> ()  [unwired: 3 in, 2 out]
                          n648 = Bundle(w853, w852) -> (w851:cluster{dbl[], dbl[]})  [unwired: 1 in]
                        }
                        frame 2 {
                          n649 = global read "Global.vi" "工位二一P"() -> (w855)
                          n650 = global read "Global.vi" "工位二—S"() -> (w856)
                          n651 = Unbundle(w863) -> (w865:dbl[], w864:dbl[])
                          n652 = call <vilib>:"Median Filter PtByPt.vi"("initialize"=w861, "rank"=w857, "x"=w859) -> ("Filtered x"=w858:dbl)  [unwired: 1 in, 1 out]
                          n653 = Build Array (concatenate)(w865, w858) -> (w868:dbl[])
                          n654 = call "Calc_Vres.vi"("S_Data in"=w856, "P_Data in"=w855) -> ("Vres"=w854:dbl)  [unwired: 7 in, 2 out]
                          n655 = call <vilib>:"Median Filter PtByPt.vi"("initialize"=w861, "rank"=w857, "x"=w854) -> ("Filtered x"=w860:dbl)  [unwired: 1 in, 1 out]
                          n656 = Build Array (concatenate)(w864, w860) -> (w867:dbl[])
                          n657 = Bundle(w868, w867) -> (w866:cluster{dbl[], dbl[]})  [unwired: 1 in]
                        }
                      }
                    }
                    n658 = local write "初始化 2"(w820) -> ()
                    n659 = local write "动优化态"(w819) -> ()
                  }
                }
                n660 = call "浮动通知.vi"("通知内容"="动态复检" ("Status")) -> ()  [unwired: 11 in]
                n661 = local read "initialize 2"() -> (w751:bool)
                n662 = case shown="默认" 0 {
                  tunnel: [w869 FALSE ("initialize 2")] -> w750
                  tunnel: w751 -> [w869 _]
                  frame Default {
                  }
                  frame 0 {
                  }
                }
                n663 = local write "选项卡控件"(enum32{"工位二程序复检", "工位二动态复检"}."工位二动态复检" ("选项卡控件")) -> ()
                n664 = local write "initialize 2"(w750) -> ()
              }
              frame 501 {
                n665 = global read "Global.vi" "动态优化完成"() -> (w871:bool)
                n666 = case shown="真" w871 {
                  frame False {
                    n667 = call "传感器数据.vi"() -> ("传感器读数"=w884:T6)  [unwired: 11 in]
                    n668 = Unbundle By Name(w884) -> ("工位二驱动伺服位移"=w879:sgl)
                    n669 = local read "动优化态前"() -> (w885:cluster{dbl[], dbl[]}[])
                    n670 = local read "初始化 3"() -> (w883:bool[])
                    n671 = for {
                      tunnel: [w892] -> w880 mode=indexing
                      tunnel: w879 -> [w891]
                      tunnel: w885 -> [w890] mode=indexing
                      tunnel: w883 -> [w888] mode=indexing
                      tunnel: [w887] -> w882 mode=indexing
                      i -> [w889]
                      n672 = case shown="5" w889 {
                        tunnel: [w894 w902 w912 w925 w938] -> w892
                        tunnel: w891 -> [_ w895 w905 w917 w932]
                        tunnel: w890 -> [w894 w899 w909 w922 w935]
                        tunnel: w888 -> [w893 w897 w908 w921 w934]
                        tunnel: [w893 FALSE ("布尔") FALSE ("布尔") FALSE ("布尔") FALSE ("布尔")] -> w887
                        tunnel: 4 ("rank") -> [_ _ _ w915 w930]
                        frame Default {
                        }
                        frame 4 {
                          n673 = call <vilib>:"Median Filter PtByPt.vi"("initialize"=w897) -> ()  [unwired: 3 in, 2 out]
                          n674 = Unbundle(w899) -> (w901:dbl[], w900:dbl[])
                          n675 = global read "Global.vi" "工位二T1"() -> (w896:dbl)
                          n676 = Build Array (concatenate)(w901, w895) -> (w904:dbl[])
                          n677 = call <vilib>:"Median Filter PtByPt.vi"("initialize"=w897) -> ()  [unwired: 3 in, 2 out]
                          n678 = Build Array (concatenate)(w900, w896) -> (w903:dbl[])
                          n679 = Bundle(w904, w903) -> (w902:cluster{dbl[], dbl[]})  [unwired: 1 in]
                        }
                        frame 5 {
                          n680 = Unbundle(w909) -> (w911:dbl[], w910:dbl[])
                          n681 = call <vilib>:"Median Filter PtByPt.vi"("initialize"=w908) -> ()  [unwired: 3 in, 2 out]
                          n682 = global read "Global.vi" "工位二T2"() -> (w906:dbl)
                          n683 = Build Array (concatenate)(w911, w905) -> (w914:dbl[])
                          n684 = call <vilib>:"Median Filter PtByPt.vi"("initialize"=w908) -> ()  [unwired: 3 in, 2 out]
                          n685 = Build Array (concatenate)(w910, w906) -> (w913:dbl[])
                          n686 = Bundle(w914, w913) -> (w912:cluster{dbl[], dbl[]})  [unwired: 1 in]
                        }
                        frame 6 {
                          n687 = call <vilib>:"Median Filter PtByPt.vi"("initialize"=w921, "rank"=w915, "x"=w917) -> ("Filtered x"=w916:dbl)  [unwired: 1 in, 1 out]
                          n688 = Unbundle(w922) -> (w924:dbl[], w923:dbl[])
                          n689 = global read "Global.vi" "工位一P"() -> (w919:dbl)
                          n690 = Build Array (concatenate)(w924, w916) -> (w927:dbl[])
                          n691 = call <vilib>:"Median Filter PtByPt.vi"("initialize"=w921, "rank"=w915, "x"=w919) -> ("Filtered x"=w918:dbl)  [unwired: 1 in, 1 out]
                          n692 = Build Array (concatenate)(w923, w918) -> (w926:dbl[])
                          n693 = Bundle(w927, w926) -> (w925:cluster{dbl[], dbl[]})  [unwired: 1 in]
                        }
                        frame 7 {
                          n694 = call <vilib>:"Median Filter PtByPt.vi"("initialize"=w934, "rank"=w930, "x"=w932) -> ("Filtered x"=w931:dbl)  [unwired: 1 in, 1 out]
                          n695 = Unbundle(w935) -> (w937:dbl[], w936:dbl[])
                          n696 = global read "Global.vi" "工位一S"() -> (w928:dbl)
                          n697 = Build Array (concatenate)(w937, w931) -> (w940:dbl[])
                          n698 = call <vilib>:"Median Filter PtByPt.vi"("initialize"=w934, "rank"=w930, "x"=w928) -> ("Filtered x"=w929:dbl)  [unwired: 1 in, 1 out]
                          n699 = Build Array (concatenate)(w936, w929) -> (w939:dbl[])
                          n700 = Bundle(w940, w939) -> (w938:cluster{dbl[], dbl[]})  [unwired: 1 in]
                        }
                      }
                    }
                    n701 = local write "初始化 3"(w882) -> ()
                    n702 = local write "动优化态前"(w880) -> ()
                    n703 = call "VRES值.vi"("XY"=w880, "索引1"=6, "索引2"=7) -> ("XY图 2"=w881:cluster{dbl[], dbl[]}[])  [unwired: 16 in]
                    n704 = Index Array(array=w881, index=8 ("索引")) -> (element=→"vRES_cCW":cluster{dbl[], dbl[]})
                  }
                  frame True {
                    n705 = call "传感器数据.vi"() -> ("传感器读数"=w945:T6)  [unwired: 11 in]
                    n706 = Unbundle By Name(w945) -> ("工位二驱动伺服位移"=w941:sgl)
                    n707 = local read "动优化态"() -> (w946:cluster{dbl[], dbl[]}[])
                    n708 = local read "初始化 2"() -> (w944:bool[])
                    n709 = for {
                      tunnel: [w953] -> w942 mode=indexing
                      tunnel: w941 -> [w952]
                      tunnel: w946 -> [w951] mode=indexing
                      tunnel: w944 -> [w949] mode=indexing
                      tunnel: [w948] -> w943 mode=indexing
                      i -> [w950]
                      n710 = case shown="5" w950 {
                        tunnel: [w955 w963 w973 w988] -> w953
                        tunnel: w952 -> [_ w956 w966 w981]
                        tunnel: w951 -> [w955 w960 w970 w985]
                        tunnel: w949 -> [w954 w958 w969 w984]
                        tunnel: [w954 FALSE ("布尔") FALSE ("布尔") FALSE ("布尔")] -> w948
                        tunnel: 4 ("rank") -> [_ _ _ w979]
                        frame Default {
                        }
                        frame 3 {
                          n711 = call <vilib>:"Median Filter PtByPt.vi"("initialize"=w958) -> ()  [unwired: 3 in, 2 out]
                          n712 = Unbundle(w960) -> (w962:dbl[], w961:dbl[])
                          n713 = global read "Global.vi" "工位二T1"() -> (w957:dbl)
                          n714 = Build Array (concatenate)(w962, w956) -> (w965:dbl[])
                          n715 = call <vilib>:"Median Filter PtByPt.vi"("initialize"=w958) -> ()  [unwired: 3 in, 2 out]
                          n716 = Build Array (concatenate)(w961, w957) -> (w964:dbl[])
                          n717 = Bundle(w965, w964) -> (w963:cluster{dbl[], dbl[]})  [unwired: 1 in]
                        }
                        frame 4 {
                          n718 = Unbundle(w970) -> (w972:dbl[], w971:dbl[])
                          n719 = call <vilib>:"Median Filter PtByPt.vi"("initialize"=w969) -> ()  [unwired: 3 in, 2 out]
                          n720 = global read "Global.vi" "工位二T2"() -> (w967:dbl)
                          n721 = Build Array (concatenate)(w972, w966) -> (w975:dbl[])
                          n722 = call <vilib>:"Median Filter PtByPt.vi"("initialize"=w969) -> ()  [unwired: 3 in, 2 out]
                          n723 = Build Array (concatenate)(w971, w967) -> (w974:dbl[])
                          n724 = Bundle(w975, w974) -> (w973:cluster{dbl[], dbl[]})  [unwired: 1 in]
                        }
                        frame 5 {
                          n725 = global read "Global.vi" "工位二一P"() -> (w977)
                          n726 = global read "Global.vi" "工位二—S"() -> (w978)
                          n727 = call <vilib>:"Median Filter PtByPt.vi"("initialize"=w984, "rank"=w979, "x"=w981) -> ("Filtered x"=w980:dbl)  [unwired: 1 in, 1 out]
                          n728 = Unbundle(w985) -> (w987:dbl[], w986:dbl[])
                          n729 = Build Array (concatenate)(w987, w980) -> (w990:dbl[])
                          n730 = call "Calc_Vres.vi"("S_Data in"=w978, "P_Data in"=w977) -> ("Vres"=w976:dbl)  [unwired: 7 in, 2 out]
                          n731 = call <vilib>:"Median Filter PtByPt.vi"("initialize"=w984, "rank"=w979, "x"=w976) -> ("Filtered x"=w982:dbl)  [unwired: 1 in, 1 out]
                          n732 = Build Array (concatenate)(w986, w982) -> (w989:dbl[])
                          n733 = Bundle(w990, w989) -> (w988:cluster{dbl[], dbl[]})  [unwired: 1 in]
                        }
                      }
                    }
                    n734 = local write "初始化 2"(w943) -> ()
                    n735 = local write "动优化态"(w942) -> ()
                  }
                }
                n736 = local read "initialize"() -> (w874:bool)
                n737 = for {
                  N: 5 -> [_]
                  tunnel: w874 -> [w992]
                  tunnel: [w993] -> w873
                  i -> [w991]
                  n738 = case shown="0" w991 {
                    tunnel: [w994 FALSE ("initialize")] -> w993
                    tunnel: w992 -> [w994 _]
                    frame Default {
                    }
                    frame 0 {
                    }
                  }
                }
                n739 = local write "initialize"(w873) -> ()
              }
              frame 502 {
                n740 = global read "Global.vi" "动态优化完成"() -> (w996:bool)
                n741 = case shown="假" w996 {
                  frame False {
                    n742 = stacked-sequence {
                      frame #0 {
                        n743 = local read "动优化态前"() -> (w997:cluster{dbl[], dbl[]}[])
                        n744 = for {
                          tunnel: w997 -> [w998] mode=indexing
                          i -> [w999]
                          n745 = Unbundle(w998) -> (w1000:dbl[])  [unwired: 1 out]
                          n746 = case shown="0" w999 {
                            tunnel: w1000 -> [_ w1001 w1002 w1003 w1004 w1005 w1006 w1007 w1008]
                            frame Default {
                            }
                            frame 0 {
                              n747 = local write "T1_CW"(w1001) -> ()
                            }
                            frame 1 {
                              n748 = local write "T2_CW"(w1002) -> ()
                            }
                            frame 2 {
                              n749 = local write "P_CW"(w1003) -> ()
                            }
                            frame 3 {
                              n750 = local write "S_CW"(w1004) -> ()
                            }
                            frame 4 {
                              n751 = local write "T1_CCw"(w1005) -> ()
                            }
                            frame 5 {
                              n752 = local write "T2_CCw"(w1006) -> ()
                            }
                            frame 6 {
                              n753 = local write "P_CCw"(w1007) -> ()
                            }
                            frame 7 {
                              n754 = local write "S_CCw"(w1008) -> ()
                            }
                          }
                        }
                      }
                      frame #1 {
                        n755 = local read "T1_CCw"() -> (w1013:dbl[])
                        n756 = local read "T2_CCw"() -> (w1015:dbl[])
                        n757 = local read "T1_CW"() -> (w1011:dbl[])
                        n758 = local read "T2_CW"() -> (w1014:dbl[])
                        n759 = Build Array(w1014, w1015) -> (w1016:dbl[][])
                        n760 = local read "SENSOR"() -> (w1017:T1)
                        n761 = call-poly <userlib>:"MGI Average.vi"("Double[][]"=w1016, "Ignore NaN? (F)"=TRUE) -> ("Average"=w1019:dbl)
                        n762 = Build Array(w1011, w1013) -> (w1012:dbl[][])
                        n763 = local read "P_CCw"() -> (w1020:dbl[])
                        n764 = local read "S_CCw"() -> (w1022:dbl[])
                        n765 = local read "S_CW"() -> (w1023:dbl[])
                        n766 = local read "P_CW"() -> (w1021:dbl[])
                        n767 = call-poly <userlib>:"MGI Average.vi"("Double[][]"=w1012, "Ignore NaN? (F)"=TRUE) -> ("Average"=w1018:dbl)
                        n768 = call "动态优化.vi"("S_CCw"=w1022, "S_Cw"=w1023, "P_CCw"=w1020, "SENSOR"=w1017, "P_Cw"=w1021, "T2_AV(%)"=w1019, "T1_AV(%)"=w1018) -> ("OK？"=w1024:bool)  [unwired: 4 in]
                        n769 = case shown="真" w1024 {
                          selector: w1024 -> [_ w1032]
                          frame False {
                          }
                          frame True {
                            n770 = global read "Global.vi" "8点复测"() -> (w1028:bool)
                            n771 = global read "Global.vi" "动态优化复测"() -> (w1031:bool)
                            n772 = global write "Global.vi" "动态优化完成"(w1032) -> ()
                            n773 = Select(t="动态优化", s=w1031, f="复测") -> (s? t:f=w1027:string)
                            n774 = Select(t=w1027, s=w1028, f="复测判定") -> (s? t:f=w1025:string)
                            n775 = local write "STEP"(w1025) -> ()
                          }
                        }
                      }
                    }
                  }
                  frame True {
                    w1037 = FALSE ("工位二占空比采集")
                    n776 = local read "动优化态"() -> (w1038:cluster{dbl[], dbl[]}[])
                    n777 = for {
                      tunnel: w1038 -> [w1039] mode=indexing
                      i -> [w1040]
                      n778 = Unbundle(w1039) -> (w1041:dbl[])  [unwired: 1 out]
                      n779 = case shown="0" w1040 {
                        tunnel: w1041 -> [_ w1042 w1043 _ w1045 w1046 _]
                        tunnel: w1039 -> [_ _ _ w1044 _ _ w1047]
                        frame Default {
                        }
                        frame 0 {
                          n780 = local write "T1_CW"(w1042) -> ()
                        }
                        frame 1 {
                          n781 = local write "T2_CW"(w1043) -> ()
                        }
                        frame 2 {
                          n782 = local write "VRES_cW"(w1044) -> ()
                        }
                        frame 3 {
                          n783 = local write "T1_CCw"(w1045) -> ()
                        }
                        frame 4 {
                          n784 = local write "T2_CCw"(w1046) -> ()
                        }
                        frame 5 {
                          n785 = local write "vRES_cCW"(w1047) -> ()
                        }
                      }
                    }
                    n786 = global write "Global.vi" "P/S采集 2"(w1037) -> ()
                    n787 = global write "Global.vi" "工位二占空比采集"(w1037) -> ()
                    n788 = global read "Global.vi" "8点复测"() -> (w1036:bool)
                    n789 = Select(t="复测", s=w1036, f="复测判定") -> (s? t:f=w1034:string)
                    n790 = local write "STEP"(w1034) -> ()
                  }
                }
              }
              frame 505 {
                w1048 = TRUE ("initialize")
                n791 = local write "initialize"(w1048) -> ()
                n792 = local write "initialize 2"(w1048) -> ()
              }
              frame 511 {
                n793 = stacked-sequence {
                  frame #0 {
                    n794 = Wait (ms)(milliseconds to wait=u32 500 ("等待时间（毫秒）")) -> ()  [unwired: 1 out]
                  }
                  frame #1 {
                    w1059 = 10171 items=["上升"=10280, "下降"=10171] ("starting edge2")
                    w1058 = 10280 items=["上升"=10280, "下降"=10171] ("starting edge1")
                    w1060 = 10171 items=["上升"=10280, "下降"=10171] ("starting edge2")
                    w1061 = 10280 items=["上升"=10280, "下降"=10171] ("starting edge1")
                    w1068 = 10171 items=["上升"=10280, "下降"=10171] ("starting edge")
                    w1070 = 10171 items=["上升"=10280, "下降"=10171] ("starting edge")
                    w1069 = 10280 items=["上升"=10280, "下降"=10171] ("starting edge")
                    w1071 = 10280 items=["上升"=10280, "下降"=10171] ("starting edge")
                    n795 = local read "VRES_cW"() -> (w1067:cluster{dbl[], dbl[]})
                    n796 = Unbundle(w1067) -> (w1065:dbl[], w1064:dbl[])
                    n797 = call "占空比测量.vi"("计数器"=tag "Dev2/ctr1", "starting edge1"=w1071, "starting edge2"=w1070) -> ("占空比2(%)"=w1074:dbl)  [unwired: 4 in, 3 out]
                    n798 = call "占空比测量.vi"("计数器"=tag "Dev2/ctr0", "starting edge1"=w1069, "starting edge2"=w1068) -> ("占空比(%)"=w1073:dbl)  [unwired: 4 in, 3 out]
                    n799 = Threshold 1D Array(2:90.0 ("分数索引或x"), 3:w1065) -> (0:w1063:dbl)  [unwired: 1 in]
                    n800 = call "占空比测量.vi"("计数器"=tag "Dev2/ctr2", "starting edge1"=w1061, "starting edge2"=w1060) -> ("占空比2(%)"=w1056:dbl)  [unwired: 4 in, 3 out]
                    n801 = call "占空比测量.vi"("计数器"=tag "Dev2/ctr3", "starting edge1"=w1058, "starting edge2"=w1059) -> ("占空比2(%)"=w1055:dbl)  [unwired: 4 in, 3 out]
                    n802 = call "Calc_Vres.vi"("S_Data in"=w1073, "P_Data in"=w1074) -> ("Vres"=w1053:dbl)  [unwired: 7 in, 2 out]
                    n803 = Interpolate 1D Array(1:w1063, 2:w1064) -> (0:w1051:dbl)
                    n804 = Subtract(x=w1056, y=w1055) -> (x-y=→"T1-T2_90°":dbl)
                    n805 = Max & Min(x=w1051, y=w1053) -> (max(x,y)=w1052:dbl)  [unwired: 1 out]
                    n806 = local write "Vres_90°"(w1052) -> ()
                  }
                  frame #2 {
                    n807 = call "设备状态.vi"("枚举"=enum16{"Read", "Write"}."Write", "工位"=enum16{"工位一", "工位二"}."工位二", "Status_Write"=i16 512) -> ()  [unwired: 8 in, 1 out]
                  }
                }
                n808 = call "浮动通知.vi"("通知内容"="正向复测！" ("Status")) -> ()  [unwired: 11 in]
              }
              frame 513 {
                n809 = stacked-sequence {
                  frame #0 {
                    n810 = Wait (ms)(milliseconds to wait=u32 500 ("等待时间（毫秒）")) -> ()  [unwired: 1 out]
                  }
                  frame #1 {
                    w1088 = 10171 items=["上升"=10280, "下降"=10171] ("starting edge2")
                    w1087 = 10280 items=["上升"=10280, "下降"=10171] ("starting edge1")
                    w1089 = 10171 items=["上升"=10280, "下降"=10171] ("starting edge2")
                    w1090 = 10280 items=["上升"=10280, "下降"=10171] ("starting edge1")
                    w1097 = 10171 items=["上升"=10280, "下降"=10171] ("starting edge")
                    w1098 = 10280 items=["上升"=10280, "下降"=10171] ("starting edge")
                    w1099 = 10171 items=["上升"=10280, "下降"=10171] ("starting edge")
                    w1100 = 10280 items=["上升"=10280, "下降"=10171] ("starting edge")
                    n811 = local read "VRES_cW"() -> (w1096:cluster{dbl[], dbl[]})
                    n812 = Unbundle(w1096) -> (w1094:dbl[], w1093:dbl[])
                    n813 = call "占空比测量.vi"("计数器"=tag "Dev2/ctr1", "starting edge1"=w1100, "starting edge2"=w1099) -> ("占空比2(%)"=w1102:dbl)  [unwired: 4 in, 3 out]
                    n814 = call "占空比测量.vi"("计数器"=tag "Dev2/ctr0", "starting edge1"=w1098, "starting edge2"=w1097) -> ("占空比(%)"=w1101:dbl)  [unwired: 4 in, 3 out]
                    n815 = Threshold 1D Array(2:180.0 ("分数索引或x"), 3:w1094) -> (0:w1092:dbl)  [unwired: 1 in]
                    n816 = call "Calc_Vres.vi"("S_Data in"=w1101, "P_Data in"=w1102) -> ("Vres"=w1081:dbl)  [unwired: 7 in, 2 out]
                    n817 = Interpolate 1D Array(1:w1092, 2:w1093) -> (0:w1080:dbl)
                    n818 = call "占空比测量.vi"("计数器"=tag "Dev2/ctr2", "starting edge1"=w1090, "starting edge2"=w1089) -> ("占空比2(%)"=w1085:dbl)  [unwired: 4 in, 3 out]
                    n819 = call "占空比测量.vi"("计数器"=tag "Dev2/ctr3", "starting edge1"=w1087, "starting edge2"=w1088) -> ("占空比2(%)"=w1084:dbl)  [unwired: 4 in, 3 out]
                    n820 = Subtract(x=w1085, y=w1084) -> (x-y=→"T1-T2_180°":dbl)
                    n821 = Max & Min(x=w1080, y=w1081) -> (max(x,y)=w1082:dbl)  [unwired: 1 out]
                    n822 = local write "Vres_180°"(w1082) -> ()
                  }
                  frame #2 {
                    n823 = call "设备状态.vi"("枚举"=enum16{"Read", "Write"}."Write", "工位"=enum16{"工位一", "工位二"}."工位二", "Status_Write"=i16 514) -> ()  [unwired: 8 in, 1 out]
                  }
                }
              }
              frame 515 {
                n824 = stacked-sequence {
                  frame #0 {
                    n825 = Wait (ms)(milliseconds to wait=u32 500 ("等待时间（毫秒）")) -> ()  [unwired: 1 out]
                  }
                  frame #1 {
                    w1117 = 10171 items=["上升"=10280, "下降"=10171] ("starting edge2")
                    w1116 = 10280 items=["上升"=10280, "下降"=10171] ("starting edge1")
                    w1118 = 10171 items=["上升"=10280, "下降"=10171] ("starting edge2")
                    w1119 = 10280 items=["上升"=10280, "下降"=10171] ("starting edge1")
                    w1126 = 10171 items=["上升"=10280, "下降"=10171] ("starting edge")
                    w1127 = 10280 items=["上升"=10280, "下降"=10171] ("starting edge")
                    w1128 = 10171 items=["上升"=10280, "下降"=10171] ("starting edge")
                    w1129 = 10280 items=["上升"=10280, "下降"=10171] ("starting edge")
                    n826 = local read "VRES_cW"() -> (w1125:cluster{dbl[], dbl[]})
                    n827 = Unbundle(w1125) -> (w1123:dbl[], w1122:dbl[])
                    n828 = call "占空比测量.vi"("计数器"=tag "Dev2/ctr1", "starting edge1"=w1129, "starting edge2"=w1128) -> ("占空比2(%)"=w1131:dbl)  [unwired: 4 in, 3 out]
                    n829 = call "占空比测量.vi"("计数器"=tag "Dev2/ctr0", "starting edge1"=w1127, "starting edge2"=w1126) -> ("占空比(%)"=w1130:dbl)  [unwired: 4 in, 3 out]
                    n830 = Threshold 1D Array(2:270.0 ("分数索引或x"), 3:w1123) -> (0:w1121:dbl)  [unwired: 1 in]
                    n831 = call "Calc_Vres.vi"("S_Data in"=w1130, "P_Data in"=w1131) -> ("Vres"=w1109:dbl)  [unwired: 7 in, 2 out]
                    n832 = call "占空比测量.vi"("计数器"=tag "Dev2/ctr2", "starting edge1"=w1119, "starting edge2"=w1118) -> ("占空比2(%)"=w1114:dbl)  [unwired: 4 in, 3 out]
                    n833 = call "占空比测量.vi"("计数器"=tag "Dev2/ctr3", "starting edge1"=w1116, "starting edge2"=w1117) -> ("占空比2(%)"=w1113:dbl)  [unwired: 4 in, 3 out]
                    n834 = Interpolate 1D Array(1:w1121, 2:w1122) -> (0:w1110:dbl)
                    n835 = Subtract(x=w1114, y=w1113) -> (x-y=→"T1-T2_270°":dbl)
                    n836 = Max & Min(x=w1110, y=w1109) -> (max(x,y)=w1111:dbl)  [unwired: 1 out]
                    n837 = local write "Vres_270°"(w1111) -> ()
                  }
                  frame #2 {
                    n838 = call "设备状态.vi"("枚举"=enum16{"Read", "Write"}."Write", "工位"=enum16{"工位一", "工位二"}."工位二", "Status_Write"=i16 516) -> ()  [unwired: 8 in, 1 out]
                  }
                }
              }
              frame 517 {
                n839 = stacked-sequence {
                  frame #0 {
                    n840 = Wait (ms)(milliseconds to wait=u32 500 ("等待时间（毫秒）")) -> ()  [unwired: 1 out]
                  }
                  frame #1 {
                    w1146 = 10171 items=["上升"=10280, "下降"=10171] ("starting edge2")
                    w1145 = 10280 items=["上升"=10280, "下降"=10171] ("starting edge1")
                    w1147 = 10171 items=["上升"=10280, "下降"=10171] ("starting edge2")
                    w1148 = 10280 items=["上升"=10280, "下降"=10171] ("starting edge1")
                    w1155 = 10171 items=["上升"=10280, "下降"=10171] ("starting edge")
                    w1156 = 10280 items=["上升"=10280, "下降"=10171] ("starting edge")
                    w1157 = 10171 items=["上升"=10280, "下降"=10171] ("starting edge")
                    w1158 = 10280 items=["上升"=10280, "下降"=10171] ("starting edge")
                    n841 = local read "VRES_cW"() -> (w1154:cluster{dbl[], dbl[]})
                    n842 = Unbundle(w1154) -> (w1152:dbl[], w1151:dbl[])
                    n843 = call "占空比测量.vi"("计数器"=tag "Dev2/ctr1", "starting edge1"=w1158, "starting edge2"=w1157) -> ("占空比2(%)"=w1160:dbl)  [unwired: 4 in, 3 out]
                    n844 = call "占空比测量.vi"("计数器"=tag "Dev2/ctr0", "starting edge1"=w1156, "starting edge2"=w1155) -> ("占空比(%)"=w1159:dbl)  [unwired: 4 in, 3 out]
                    n845 = Threshold 1D Array(2:360.0 ("分数索引或x"), 3:w1152) -> (0:w1150:dbl)  [unwired: 1 in]
                    n846 = call "Calc_Vres.vi"("S_Data in"=w1159, "P_Data in"=w1160) -> ("Vres"=w1138:dbl)  [unwired: 7 in, 2 out]
                    n847 = call "占空比测量.vi"("计数器"=tag "Dev2/ctr2", "starting edge1"=w1148, "starting edge2"=w1147) -> ("占空比2(%)"=w1143:dbl)  [unwired: 4 in, 3 out]
                    n848 = call "占空比测量.vi"("计数器"=tag "Dev2/ctr3", "starting edge1"=w1145, "starting edge2"=w1146) -> ("占空比2(%)"=w1142:dbl)  [unwired: 4 in, 3 out]
                    n849 = Interpolate 1D Array(1:w1150, 2:w1151) -> (0:w1139:dbl)
                    n850 = Subtract(x=w1143, y=w1142) -> (x-y=→"T1-T2_360°":dbl)
                    n851 = Max & Min(x=w1139, y=w1138) -> (max(x,y)=w1140:dbl)  [unwired: 1 out]
                    n852 = local write "Vres_360°"(w1140) -> ()
                  }
                  frame #2 {
                    n853 = call "设备状态.vi"("枚举"=enum16{"Read", "Write"}."Write", "工位"=enum16{"工位一", "工位二"}."工位二", "Status_Write"=i16 520) -> ()  [unwired: 8 in, 1 out]
                  }
                }
              }
              frame 521 {
                n854 = stacked-sequence {
                  frame #0 {
                    n855 = Wait (ms)(milliseconds to wait=u32 500 ("等待时间（毫秒）")) -> ()  [unwired: 1 out]
                  }
                  frame #1 {
                    w1176 = 10171 items=["上升"=10280, "下降"=10171] ("starting edge2")
                    w1175 = 10280 items=["上升"=10280, "下降"=10171] ("starting edge1")
                    w1177 = 10171 items=["上升"=10280, "下降"=10171] ("starting edge2")
                    w1178 = 10280 items=["上升"=10280, "下降"=10171] ("starting edge1")
                    w1187 = 10171 items=["上升"=10280, "下降"=10171] ("starting edge")
                    w1188 = 10280 items=["上升"=10280, "下降"=10171] ("starting edge")
                    w1189 = 10171 items=["上升"=10280, "下降"=10171] ("starting edge")
                    w1190 = 10280 items=["上升"=10280, "下降"=10171] ("starting edge")
                    n856 = local read "vRES_cCW"() -> (w1186:cluster{dbl[], dbl[]})
                    n857 = Unbundle(w1186) -> (w1183:dbl[], w1181:dbl[])
                    n858 = call "占空比测量.vi"("计数器"=tag "Dev2/ctr1", "starting edge1"=w1190, "starting edge2"=w1189) -> ("占空比2(%)"=w1192:dbl)  [unwired: 4 in, 3 out]
                    n859 = call "占空比测量.vi"("计数器"=tag "Dev2/ctr0", "starting edge1"=w1188, "starting edge2"=w1187) -> ("占空比(%)"=w1191:dbl)  [unwired: 4 in, 3 out]
                    n860 = Reverse 1D Array(array=w1183) -> (reversed array=w1182:dbl[])
                    n861 = Threshold 1D Array(2:315.0 ("分数索引或x"), 3:w1182) -> (0:w1184:dbl)  [unwired: 1 in]
                    n862 = call "Calc_Vres.vi"("S_Data in"=w1191, "P_Data in"=w1192) -> ("Vres"=w1168:dbl)  [unwired: 7 in, 2 out]
                    n863 = Reverse 1D Array(array=w1181) -> (reversed array=w1180:dbl[])
                    n864 = call "占空比测量.vi"("计数器"=tag "Dev2/ctr4", "starting edge1"=w1178, "starting edge2"=w1177) -> ("占空比2(%)"=w1173:dbl)  [unwired: 4 in, 3 out]
                    n865 = call "占空比测量.vi"("计数器"=tag "Dev2/ctr5", "starting edge1"=w1175, "starting edge2"=w1176) -> ("占空比2(%)"=w1172:dbl)  [unwired: 4 in, 3 out]
                    n866 = Interpolate 1D Array(1:w1184, 2:w1180) -> (0:w1169:dbl)
                    n867 = Subtract(x=w1173, y=w1172) -> (x-y=→"T1-T2_315°":dbl)
                    n868 = Max & Min(x=w1168, y=w1169) -> (max(x,y)=w1170:dbl)  [unwired: 1 out]
                    n869 = local write "Vres_315°"(w1170) -> ()
                  }
                  frame #2 {
                    n870 = call "设备状态.vi"("枚举"=enum16{"Read", "Write"}."Write", "工位"=enum16{"工位一", "工位二"}."工位二", "Status_Write"=i16 522) -> ()  [unwired: 8 in, 1 out]
                  }
                }
                n871 = call "浮动通知.vi"("通知内容"="逆向复测！" ("Status")) -> ()  [unwired: 11 in]
              }
              frame 523 {
                n872 = stacked-sequence {
                  frame #0 {
                    n873 = Wait (ms)(milliseconds to wait=u32 500 ("等待时间（毫秒）")) -> ()  [unwired: 1 out]
                  }
                  frame #1 {
                    w1207 = 10171 items=["上升"=10280, "下降"=10171] ("starting edge2")
                    w1206 = 10280 items=["上升"=10280, "下降"=10171] ("starting edge1")
                    w1208 = 10171 items=["上升"=10280, "下降"=10171] ("starting edge2")
                    w1209 = 10280 items=["上升"=10280, "下降"=10171] ("starting edge1")
                    w1218 = 10171 items=["上升"=10280, "下降"=10171] ("starting edge")
                    w1219 = 10280 items=["上升"=10280, "下降"=10171] ("starting edge")
                    w1220 = 10171 items=["上升"=10280, "下降"=10171] ("starting edge")
                    w1221 = 10280 items=["上升"=10280, "下降"=10171] ("starting edge")
                    n874 = local read "vRES_cCW"() -> (w1217:cluster{dbl[], dbl[]})
                    n875 = Unbundle(w1217) -> (w1214:dbl[], w1212:dbl[])
                    n876 = Reverse 1D Array(array=w1214) -> (reversed array=w1213:dbl[])
                    n877 = call "占空比测量.vi"("计数器"=tag "Dev2/ctr1", "starting edge1"=w1221, "starting edge2"=w1220) -> ("占空比2(%)"=w1223:dbl)  [unwired: 4 in, 3 out]
                    n878 = call "占空比测量.vi"("计数器"=tag "Dev2/ctr0", "starting edge1"=w1219, "starting edge2"=w1218) -> ("占空比(%)"=w1222:dbl)  [unwired: 4 in, 3 out]
                    n879 = Threshold 1D Array(2:225.0 ("分数索引或x"), 3:w1213) -> (0:w1215:dbl)  [unwired: 1 in]
                    n880 = Reverse 1D Array(array=w1212) -> (reversed array=w1211:dbl[])
                    n881 = call "Calc_Vres.vi"("S_Data in"=w1222, "P_Data in"=w1223) -> ("Vres"=w1199:dbl)  [unwired: 7 in, 2 out]
                    n882 = Interpolate 1D Array(1:w1215, 2:w1211) -> (0:w1200:dbl)
                    n883 = call "占空比测量.vi"("计数器"=tag "Dev2/ctr2", "starting edge1"=w1209, "starting edge2"=w1208) -> ("占空比2(%)"=w1204:dbl)  [unwired: 4 in, 3 out]
                    n884 = call "占空比测量.vi"("计数器"=tag "Dev2/ctr3", "starting edge1"=w1206, "starting edge2"=w1207) -> ("占空比2(%)"=w1203:dbl)  [unwired: 4 in, 3 out]
                    n885 = Subtract(x=w1204, y=w1203) -> (x-y=→"T1-T2_225°":dbl)
                    n886 = Max & Min(x=w1200, y=w1199) -> (max(x,y)=w1201:dbl)  [unwired: 1 out]
                    n887 = local write "Vres_225°"(w1201) -> ()
                  }
                  frame #2 {
                    n888 = call "设备状态.vi"("枚举"=enum16{"Read", "Write"}."Write", "工位"=enum16{"工位一", "工位二"}."工位二", "Status_Write"=i16 524) -> ()  [unwired: 8 in, 1 out]
                  }
                }
              }
              frame 525 {
                n889 = stacked-sequence {
                  frame #0 {
                    n890 = Wait (ms)(milliseconds to wait=u32 500 ("等待时间（毫秒）")) -> ()  [unwired: 1 out]
                  }
                  frame #1 {
                    w1238 = 10171 items=["上升"=10280, "下降"=10171] ("starting edge2")
                    w1237 = 10280 items=["上升"=10280, "下降"=10171] ("starting edge1")
                    w1239 = 10171 items=["上升"=10280, "下降"=10171] ("starting edge2")
                    w1240 = 10280 items=["上升"=10280, "下降"=10171] ("starting edge1")
                    w1249 = 10171 items=["上升"=10280, "下降"=10171] ("starting edge")
                    w1250 = 10280 items=["上升"=10280, "下降"=10171] ("starting edge")
                    w1251 = 10171 items=["上升"=10280, "下降"=10171] ("starting edge")
                    w1252 = 10280 items=["上升"=10280, "下降"=10171] ("starting edge")
                    n891 = local read "vRES_cCW"() -> (w1248:cluster{dbl[], dbl[]})
                    n892 = Unbundle(w1248) -> (w1243:dbl[], w1245:dbl[])
                    n893 = Reverse 1D Array(array=w1243) -> (reversed array=w1242:dbl[])
                    n894 = call "占空比测量.vi"("计数器"=tag "Dev2/ctr1", "starting edge1"=w1252, "starting edge2"=w1251) -> ("占空比2(%)"=w1254:dbl)  [unwired: 4 in, 3 out]
                    n895 = call "占空比测量.vi"("计数器"=tag "Dev2/ctr0", "starting edge1"=w1250, "starting edge2"=w1249) -> ("占空比(%)"=w1253:dbl)  [unwired: 4 in, 3 out]
                    n896 = Threshold 1D Array(2:135.0 ("分数索引或x"), 3:w1242) -> (0:w1246:dbl)  [unwired: 1 in]
                    n897 = Reverse 1D Array(array=w1245) -> (reversed array=w1244:dbl[])
                    n898 = call "Calc_Vres.vi"("S_Data in"=w1253, "P_Data in"=w1254) -> ("Vres"=w1231:dbl)  [unwired: 7 in, 2 out]
                    n899 = Interpolate 1D Array(1:w1246, 2:w1244) -> (0:w1230:dbl)
                    n900 = call "占空比测量.vi"("计数器"=tag "Dev2/ctr2", "starting edge1"=w1240, "starting edge2"=w1239) -> ("占空比2(%)"=w1235:dbl)  [unwired: 4 in, 3 out]
                    n901 = call "占空比测量.vi"("计数器"=tag "Dev2/ctr3", "starting edge1"=w1237, "starting edge2"=w1238) -> ("占空比2(%)"=w1234:dbl)  [unwired: 4 in, 3 out]
                    n902 = Max & Min(x=w1230, y=w1231) -> (max(x,y)=w1232:dbl)  [unwired: 1 out]
                    n903 = Subtract(x=w1235, y=w1234) -> (x-y=→"T1-T2_135°":dbl)
                    n904 = local write "Vres_135°"(w1232) -> ()
                  }
                  frame #2 {
                    n905 = call "设备状态.vi"("枚举"=enum16{"Read", "Write"}."Write", "工位"=enum16{"工位一", "工位二"}."工位二", "Status_Write"=i16 526) -> ()  [unwired: 8 in, 1 out]
                  }
                }
              }
              frame 527 {
                n906 = stacked-sequence {
                  frame #0 {
                    n907 = Wait (ms)(milliseconds to wait=u32 500 ("等待时间（毫秒）")) -> ()  [unwired: 1 out]
                  }
                  frame #1 {
                    w1267 = 10171 items=["上升"=10280, "下降"=10171] ("starting edge2")
                    w1268 = 10280 items=["上升"=10280, "下降"=10171] ("starting edge1")
                    w1264 = 10171 items=["上升"=10280, "下降"=10171] ("starting edge2")
                    w1265 = 10280 items=["上升"=10280, "下降"=10171] ("starting edge1")
                    w1280 = 10171 items=["上升"=10280, "下降"=10171] ("starting edge")
                    w1281 = 10280 items=["上升"=10280, "下降"=10171] ("starting edge")
                    w1282 = 10171 items=["上升"=10280, "下降"=10171] ("starting edge")
                    w1283 = 10280 items=["上升"=10280, "下降"=10171] ("starting edge")
                    n908 = local read "vRES_cCW"() -> (w1279:cluster{dbl[], dbl[]})
                    n909 = Unbundle(w1279) -> (w1275:dbl[], w1274:dbl[])
                    n910 = call "占空比测量.vi"("计数器"=tag "Dev2/ctr1", "starting edge1"=w1283, "starting edge2"=w1282) -> ("占空比2(%)"=w1285:dbl)  [unwired: 4 in, 3 out]
                    n911 = call "占空比测量.vi"("计数器"=tag "Dev2/ctr0", "starting edge1"=w1281, "starting edge2"=w1280) -> ("占空比(%)"=w1284:dbl)  [unwired: 4 in, 3 out]
                    n912 = Reverse 1D Array(array=w1275) -> (reversed array=w1276:dbl[])
                    n913 = call "Calc_Vres.vi"("S_Data in"=w1284, "P_Data in"=w1285) -> ("Vres"=w1262:dbl)  [unwired: 7 in, 2 out]
                    n914 = Reverse 1D Array(array=w1274) -> (reversed array=w1273:dbl[])
                    n915 = Threshold 1D Array(2:45.0 ("分数索引或x"), 3:w1276) -> (0:w1278:dbl)  [unwired: 1 in]
                    n916 = Interpolate 1D Array(1:w1278, 2:w1273) -> (0:w1261:dbl)
                    n917 = Max & Min(x=w1261, y=w1262) -> (max(x,y)=w1263:dbl)  [unwired: 1 out]
                    n918 = call "占空比测量.vi"("计数器"=tag "Dev2/ctr2", "starting edge1"=w1265, "starting edge2"=w1264) -> ("占空比2(%)"=w1272:dbl)  [unwired: 4 in, 3 out]
                    n919 = call "占空比测量.vi"("计数器"=tag "Dev2/ctr3", "starting edge1"=w1268, "starting edge2"=w1267) -> ("占空比2(%)"=w1271:dbl)  [unwired: 4 in, 3 out]
                    n920 = local write "Vres_45°"(w1263) -> ()
                    n921 = Subtract(x=w1272, y=w1271) -> (x-y=→"T1-T2_45°":dbl)
                  }
                  frame #2 {
                    n922 = local write "STEP"("复测判定") -> ()
                  }
                }
              }
              frame 530 {
              }
              frame 1024 {
                n923 = local write "STEP"("退出自动" ("STEP")) -> ()
              }
            }
          }
          frame "不合格" {
            n924 = Wait (ms)(milliseconds to wait=u32 100 ("等待时间（毫秒）")) -> ()  [unwired: 1 out]
            n925 = local write "STEP"("等待" ("STEP")) -> ()
            n926 = call "设备状态.vi"("枚举"=enum16{"Read", "Write"}."Write", "工位"=enum16{"工位一", "工位二"}."工位二", "Status_Write"=i16 400) -> ()  [unwired: 8 in, 1 out]
          }
          frame "报表" {
            n927 = stacked-sequence {
              frame #0 {
                n928 = global write "Global.vi" "计时开始"(FALSE ("计时开始")) -> ()
              }
              frame #1 {
                n929 = disable-structure shown="禁用" {
                  frame Disabled {
                    n930 = global read "Global.vi" "产品编号"() -> (w1304:string)
                    n931 = Concatenate Strings("graph\\" ("名称或相对路径"), w1304, ".hsg" ("字符串")) -> (w1305:string)
                    n932 = call <vilib>:"Application Directory.vi"() -> ("Application Directory"=w1307:path)
                    n933 = local read "动优化态前"() -> (w1311:cluster{dbl[], dbl[]}[])
                    n934 = local read "传感器复检"() -> (w1296:cluster{dbl[], dbl[]}[])
                    n935 = local read "动优化态"() -> (w1312:cluster{dbl[], dbl[]}[])
                    n936 = Build Path(base path=w1307, name or relative path=w1305) -> (appended path=w1300:path)
                    n937 = Bundle("动优化态"=w1312, "动优化态前"=w1311, "传感器复检"=w1296) -> (w1310:T9)  [unwired: 1 in]
                    n938 = Open/Create/Replace File(file path (use dialog)=w1300, operation (0:open)=T5."open or create" ("操作(0:open)")) -> (refnum out=w1298:refnum<file>, error out=w1297:errorcluster)  [unwired: 4 in, 1 out]
                    n939 = Flatten To JSON(anything=w1310, error in (no error)=w1297) -> (JSON string=w1309:string, 11:w1308:errorcluster)  [unwired: 1 in]
                    n940 = Write to Binary File(file (use dialog)=w1298, data=w1309, error in=w1308) -> (refnum out=w1301:refnum<file>, error out=w1302:errorcluster)  [unwired: 3 in, 1 out]
                    n941 = Close File(refnum=w1301, error in=w1302) -> ()  [unwired: 2 out]
                  }
                  frame Enabled {
                  }
                }
              }
              frame #2 {
                n942 = global read "Global.vi" "产品编号 2"() -> (w1315)
                n943 = call "Report.vi"("文件重命名"=TRUE, "文件名称"=w1315, "判定结果"="判定结果") -> ("RESULT_VALUE"=w1313:string)  [unwired: 7 in, 1 out]
                n944 = global read "Global.vi" "联机模式"() -> (w1317:enum16{"单机", "追溯"})
                n945 = case shown="\"追溯\"" w1317 {
                  tunnel: w1313 -> [_ w1318]
                  frame "单机", Default {
                  }
                  frame "追溯" {
                    n946 = global read "Global.vi" "Result 2"() -> (w1323)
                    n947 = property class="Tbl"(reference=w1323) -> (reference out=w1322:refnum<vi>, "Row Headers[]"=w1320:string[])  [unwired: 1 in, 1 out]
                    n948 = property class="Tbl"(reference=w1322) -> ("Value"=w1321:string[][])  [unwired: 1 in, 2 out]
                    n949 = for {
                      tunnel: w1321 -> [w1329] mode=indexing
                      tunnel: w1320 -> [w1330] mode=indexing
                      tunnel: [w1327] -> w1319 mode=indexing if=w1328
                      n950 = Index Array(array=w1329) -> (element=w1331:string)  [unwired: 1 in]
                      n951 = Build Array (concatenate)(w1330, w1329) -> (w1327:string[])
                      n952 = case shown="\"\"" w1331 {
                        tunnel: [TRUE FALSE] -> w1328
                        frame Default {
                        }
                        frame "" {
                        }
                      }
                    }
                    n953 = global read "追溯Global.vi" "DEVICE_ID"() -> (w1325:string)
                    n954 = global read "追溯Global.vi" "CODE_ID"() -> (w1324:string)
                    n955 = global read "追溯Global.vi" "USER_ID"() -> (w1326:string)
                    n956 = call "UPRESULT.vi"("DEVICE_ID"=w1325, "USER_ID"=w1326, "CODE_ID"=w1324, "RESULT_VALUE"=w1318) -> ()  [unwired: 11 in, 1 out]
                    n957 = call "UPTEST.vi"("Result"=w1319, "CODE_ID"=w1324, "DEVICE_ID"=w1325) -> ()  [unwired: 6 in, 1 out]
                  }
                }
              }
              frame #3 {
                n958 = local write "STEP"("进入自动" ("STEP")) -> ()
              }
            }
          }
        }
        n959 = global read "Global.vi" "程序关闭"() -> (w13:bool)
      }
      n960 = while {
        stop <- w1335 stop-if-true
        n961 = event shown="[5] \"传感器复检\": 鼠标按下" {
          selector: _ -> [_ _ _ _ _ _]
          dyn-events: _ -> [_ _ _ _ _ _]
          timeout: -1 -> [_ _ _ _ _ _]
          event Timeout {
            (unwired) enum32{"工位二程序复检", "工位二动态复检"}."工位二程序复检" ("选项卡控件")
            n962 = event-data() -> ()  [unwired: 1 in, 3 out]
            n963 = call "Obtain Broadcast Events for Registration.vi"() -> ("Already running?"=w1337:bool)  [unwired: 9 in, 2 out]
            n964 = case shown="真" w1337 {
              frame False {
                n965 = local write "STEP"("手动" ("STEP")) -> ()
              }
              frame True {
                n966 = call "错误代码.vi"() -> ("Status_Read"=w1339:u32)  [unwired: 11 in]
                n967 = feedback #9() -> (w1349:u32)  [unwired: 1 in]
                n968 = feedback-in #9(w1339) -> ()
                n969 = case shown="0" w1339 {
                  frame 0 {
                    n970 = global read "Global.vi" "报警图标"() -> (w1350:refnum<vi>)
                    n971 = property class="Bool"(reference=w1350, "Visible"=FALSE ("可见")) -> ()  [unwired: 1 in, 2 out]
                  }
                  frame 1, Default {
                    n972 = global read "Global.vi" "报警图标"() -> (w1353:refnum<vi>)
                    n973 = property class="Bool"(reference=w1353, "Visible"=TRUE ("可见")) -> ()  [unwired: 1 in, 2 out]
                  }
                }
                n974 = Greater Or Equal?(x=w1339, y=i16 5000) -> (x >= y?=w1347:bool)
                n975 = Less?(x=w1339, y=i16 5200) -> (x < y?=w1348:bool)
                n976 = Equal?(x=w1339, y=w1349) -> (x = y?=w1346:bool)
                n977 = global read "Global.vi" "报警图标"() -> (w1341:refnum<vi>)
                n978 = And(x=w1347, y=w1348) -> (x .and. y?=w1340:bool)
                n979 = property class="Bool"(reference=w1341, "Value"=w1340) -> ()  [unwired: 1 in, 2 out]
                n980 = Bundle By Name(cluster=errorcluster {"status"=FALSE, "code"=0, "source"=""} ("错误常量"), "status"=w1340, "code"=w1339) -> (w1345:errorcluster)
                n981 = case shown="假" w1346 {
                  tunnel: w1345 -> [w1354 _]
                  frame False {
                    n982 = call "报警处理.vi"("错误常量"=w1354) -> ()  [unwired: 9 in, 2 out]
                  }
                  frame True {
                  }
                }
              }
            }
          }
          event Menu Selection (User) {
            n983 = event-data() -> ("ItemTag"=w1355:string)  [unwired: 1 in, 2 out]
            n984 = case shown="\"真\"" w1355 {
              frame "假", Default {
              }
              frame "真" {
              }
            }
          }
          event "传感器复检": Scale Range Change {
            n985 = event-data() -> ("CtlRef"=w1356:refnum<vi>)  [unwired: 1 in]
            n986 = call "XY_conf.vi"("方式"=enum16{"写入", "读取"}."写入", "XY图引用"=w1356) -> ()  [unwired: 3 in, 1 out]
          }
          event Panel Close {
            n987 = event-data() -> ()  [unwired: 1 in, 4 out]
            n988 = global write "Global.vi" "程序关闭"(TRUE ("程序关闭")) -> ()
          }
          event "传感器复检": Mouse Enter; "传感器复检": Mouse Leave; "传感器复检": Cursor Move {
            n989 = event-data() -> ("CtlRef"=w1361:refnum<vi>, "Type"=w1359:T10)  [unwired: 1 in]
            n990 = call "CursorShow.vi"("nameShow"=TRUE, "Type"=w1359, "Graph"=w1361) -> ()  [unwired: 7 in, 2 out]
          }
          event "传感器复检": Mouse Down {
            n991 = event-data() -> ("CtlRef"=w1366:refnum<vi>, "Coords"=w1365:T11, "Type"=w1363:T10)  [unwired: 1 in]
            n992 = invoke class="XYGraph (严格)" method="Map Coords To XY"(reference=w1366, "Coords"=w1365) -> (reference out=w1364:refnum<vi>, "XY"=w1362:cluster{"X":dbl, "Y":dbl})  [unwired: 5 in, 5 out]
            n993 = call "CursorShow.vi"("游标.游标位置"=w1362, "Type"=w1363, "Graph"=w1364) -> ()  [unwired: 7 in, 2 out]
          }
        }
        n994 = global read "Global.vi" "程序关闭"() -> (w1335:bool)
      }
    }
  }
